vi "POM_PROM_ТЗЧ(3)_host.vi"() -> ()   [LabVIEW 2013]
uses:
  <instrlib>/niDMM/nidmm.llb/niDMM Resolution in Digits.ctl
  <instrlib>/niDMM/nidmm.llb/niDMM Function.ctl
  <vilib>/Analysis/baseanly.llb/Mean (DBL).vi
  <instrlib>/niDMM/nidmm.llb/niDMM Configure Measurement Digits.vi
  <vilib>/Analysis/NI_AALBase.lvlib
  <instrlib>/niDCPower/nidcpower.llb/niDCPower Measurement Type.ctl
panel:
  in  "Нагрев":bool
  in  "В ручную":bool
  in  "Напряжение Пельтье":dbl=0.03
  in  "milliseconds to wait 2":u32=40
  out "Monitor current, uA":dbl(graph)=356.9975233403966
  in  "Порог типатиристора, мА":dbl=55.0
  out "Счетчик сбоев":dbl=6.0
  out "Температура":i32=25
  out "Образец":i32=180201
  out "Сеанс":i32=5
  out "Ион":string="Проверка"
  in  "SEL simulation":bool
  out "refnum out":refnum<file>
  in  "Облучение!":bool
  out "Стабилизировано":bool=TRUE
  in  "+ V TEC для новой точки":dbl=0.11 format="%#_13g"
  in  "Вычет для \"антиразгона\"":dbl format="%#_13g"
  in  "Оставить в раб.\nрежиме":bool
  out "Boolean":bool
  in  "Num_hits_req":u64
  out "Num_hits":u64=15
  in  "Count_hits?":bool
  in  "tstab между точками, мс":u32=1
  in  "Предел тока PDext, мА":dbl=20.0
  in  "Отладка(F)/\n/Рабочий(T)":bool=TRUE
  out "TEC_current, mA":dbl=84.01255498914388
  in  "Param_Log":path=path "D:/#rkm/Фонон-4/ТермоЛазер/Фонон-4_ПОМ_ПрОМ/Прога/Updated/ThermoLaser/Logs/Проверка"
  in  "trelax":u32=35000
  out "Volt_onRes":dbl=2.4602762193630356
  out "NoStab":bool
  out "Operating Current, mA":dbl=48.79715117716259
  in  "Desirable Operating current, mA":dbl=50.0 format="%#_6f"
  in  "Up_Volt_limit":dbl=5.0
  in  "Low_Volt_limit":dbl=1.0
  out "ThRes_stabil":bool=TRUE
  out "Подстроенное напряжение\nстабилизации":dbl=0.22536355468750027
  out "ThRes value":dbl=18041.63984375
  in  "Optimum ThRes":dbl=18000.0 format="%#_6f"
  in  "Предел тока LD, мА":dbl=100.0
  in  "Предел тока ТЕС, мА":dbl=300.0
  in  "Tab Control":enum32{"Page 1", "Page 2", "Page 3", "Page 4"}(tab)=enum."Page 4"
  out "RES(U_TEC) Graph":cluster{dbl[], dbl[]}(graph)={[-0.0, 0.025, 0.05, 0.07500000000000001, 0.1, 0.125, 0.15, 0.175, 0.19999999999999998, 0.22499999999999998, 0.24999999999999997, 0.27499999999999997, 0.3, 0.325, 0.35000000000000003, 0.37500000000000006, 0.4000000000000001, 0.4250000000000001, 0.4500000000000001, 0.47500000000000014, 0.5000000000000001, 0.5250000000000001, 0.5500000000000002, 0.5750000000000002, 0.6000000000000002, 0.6250000000000002, 0.6500000000000002, 0.6750000000000003, 0.7000000000000003, 0.7250000000000003, 0.7500000000000003, 0.7750000000000004], [15319.04365234375, 15328.19267578125, 15358.49169921875, 15409.562109375, 15479.3826171875, 15563.1861328125, 15668.50888671875, 15780.12734375, 15906.40224609375, 16043.244921875, 16186.97255859375, 16341.84609375, 16507.0697265625, 16676.522265625, 16856.963671875, 17044.884375, 17239.0294921875, 17436.3736328125, 17641.744140625, 17850.8728515625, 18071.7896484375, 18291.20625, 18518.965625, 18750.4271484375, 18987.4517578125, 19230.0744140625, 19480.026171875, 19731.8517578125, 19984.940234375, 20249.54140625, 20514.206640625, 20780.055078125]}
  out "RES(I_TEC) Graph":cluster{dbl[], dbl[]}(graph)={[0.03457500435386299, 4.049114950716204, 7.9212407853678135, 11.611043015146826, 15.078954849250364, 18.53827902856892, 21.88408259580828, 25.295266856430793, 28.546483256934756, 31.60504570629327, 34.77027313644012, 37.80993408960394, 40.856486299311584, 43.94949565069024, 47.03219408159836, 50.06845592920464, 52.92926046093485, 55.95350027659507, 58.865931959242474, 61.84202368829837, 64.7802788203752, 67.60156326899994, 70.44177990185035, 73.41963022613506, 76.46974363403558, 79.22741287887104, 82.2001312992484, 85.07135997639818, 88.0785044464861, 90.98931976346292, 93.95691599392462, 96.75420696595256], [15319.04365234375, 15328.19267578125, 15358.49169921875, 15409.562109375, 15479.3826171875, 15563.1861328125, 15668.50888671875, 15780.12734375, 15906.40224609375, 16043.244921875, 16186.97255859375, 16341.84609375, 16507.0697265625, 16676.522265625, 16856.963671875, 17044.884375, 17239.0294921875, 17436.3736328125, 17641.744140625, 17850.8728515625, 18071.7896484375, 18291.20625, 18518.965625, 18750.4271484375, 18987.4517578125, 19230.0744140625, 19480.026171875, 19731.8517578125, 19984.940234375, 20249.54140625, 20514.206640625, 20780.055078125]}
  out "I_PD_Ext(I_LD) Graph":cluster{dbl[], dbl[]}(graph)={[0.0, 5.125820672560687, 10.202363077068034, 15.09070291650038, 20.026524721844005, 24.848748653112324, 29.706585438813228, 34.55255888002156, 39.41379829521783, 44.31743313126964, 49.35841653002704], [0.6213749657825949, 0.6126206411732633, 0.5986137214569519, 0.5846068013204628, 0.5933611264550083, 0.5670981505590477, 0.5355825775341941, 0.586357666360488, 0.5355825775341941, 0.5478386339632713, 0.5390843079753067]}
  out "I_PD(I_LD) Graph":cluster{dbl[], dbl[]}(graph)={[0.0, 5.125820672560687, 10.202363077068034, 15.09070291650038, 20.026524721844005, 24.848748653112324, 29.706585438813228, 34.55255888002156, 39.41379829521783, 44.31743313126964, 49.35841653002704], [0.00446055423708458, 0.1890051237296575, 1.3185992656872259, 47.69851657329127, 96.3842059718445, 145.3466946259141, 195.95923949964345, 243.1108383461833, 288.08951028622687, 334.6654470078647, 377.8655605856329]}
  out "I_pd, uA":dbl
  out "IPD(ext), mA":dbl
  out "V2(I_LD) Graph":cluster{dbl[], dbl[]}(graph)={[0.0, 5.125820672560687, 10.202363077068034, 15.09070291650038, 20.026524721844005, 24.848748653112324, 29.706585438813228, 34.55255888002156, 39.41379829521783, 44.31743313126964, 49.35841653002704], [0.0006418486043783589, 1.1699665507043246, 1.452329111789965, 1.6798119558569469, 1.9201177244634586, 2.150803801269446, 2.3862573437846697, 2.612869753183121, 2.8439823589319366, 3.0683008415602466, 3.3013683877429134]}
  out "Forward Voltage, V":dbl
  out "OP(I_LD) Graph":cluster{dbl[], dbl[]}(graph)={[0.0, 5.125820672560687, 10.202363077068034, 15.09070291650038, 20.026524721844005, 24.848748653112324, 29.706585438813228, 34.55255888002156, 39.41379829521783, 44.31743313126964, 49.35841653002704], [0.0, 0.0, 0.02, 0.74, 1.5, 2.27, 3.0300000000000002, 3.8, 4.58, 5.33, 6.119999999999999]}
  out "Ophir, mW":dbl
  out "Пороговый ток":dbl
  out "ExtPhotodiode Current":dbl(graph)
  out "Boolean 2":bool
  out "Сопротивление терморез-ра":dbl(graph)=16035.80078125
  out "thRes_adj":dbl=16035.80078125 format="%0.2f"
  in  "Source-Ohm w8":u32=1000
  in  "Coeff_High":dbl=90000.0 format="%#_13g"
  in  "Coeff_low":dbl=20000.0 format="%#_13g"
  in  "Coeff_thr":dbl=1500.0
  out "+Voltage\nrequired":dbl=0.0008410915798611111
  out "Разница ThRes":dbl=75.6982421875
  out "Operating Current":dbl(graph)
  out "Готовы облучать":bool
  out "accommodated voltage (out)":dbl=5.873393180232852
  in  "4070_Rele_source":enum16{"S2_Ch0", "S1_Ch2"}(ring)
  in  "the upper limit for the voltage_LD":dbl=6.0
  in  "the lower limit for the voltage_LD":dbl=1.0
  in  "Start voltage_LD":dbl=2.0 format="%#.7f"
  in  "accuracy_LD":dbl=0.09999999999999999 step=0.01
  in  "Res_LD":dbl=50.0
  in  "TEC_Source":enum16{"S1_Ch2", "S2_Ch0", "S3_Ch1"}(ring)
  in  "Start voltage":dbl=0.1 format="%#.7f"
  in  "the upper limit for the voltage":dbl=0.9
  in  "the lower limit for the voltage":dbl
  in  "Точность ThRes":dbl=75.0 step=0.01
  out "Ro, Ом":dbl=15321.56484375
  in  "OphirLMMeasurementLib.ICoLMMeasurement":refnum<k7>
  out "hDevice":i32=1004
  out "Ophir_address":refnum<k7>
  in  "Power Enable":bool
  in  "4071(2)":refnum<k15>
  out "4071(2)_adress":refnum<k15>="PXI1Slot4_2 (12)" caption="4071(1)_out"
  in  "4071(1)":refnum<k15>="PXI1Slot5_2"
  out "4071(1)_adress":refnum<k15>="PXI1Slot5_2 (8)" caption="4071(1)_out"
  out "4070_address":refnum<k15>="PXI1Slot4_2 (8)" caption="4070_out"
  in  "4070":refnum<k15>="PXI1Slot6_3"
  in  "Source_3":refnum<k15>
  out "Source_3_Vcc_out":refnum<k15> caption="S_3_out"
  out "Source_2_Vcc_out":refnum<k15>="PXI1Slot6" caption="S_2_out"
  in  "Source_2":refnum<k15>="PXI1Slot3"
  out "Source_1_Vcc_out":refnum<k15>="PXI1Slot2_2" caption="S_1_out"
  in  "Source_1":refnum<k15>="PXI1Slot2_2"
  out "Прервать":bool=TRUE
  in  "milliseconds to wait":u32=2000
  in  "Шаг напр\nдля TEC, В":dbl=0.025
  in  "Начальное\nнапряжение TEC, В":dbl
  in  "кол-во точек для TEC":i32=32
  in  "stop":bool
  in  "Case":T1(ring)=enum."Quit"
  out "Выполняется":bool
  in  "Раб. режим LD":bool
  in  "Хар-ка TEC":bool
  in  "Хар-ки от I_LD":bool
  out "Status:":string="IDLE"
  out "Подстроенный ток, mA":dbl=48.878464927379845
  in  "Шаг, мА":dbl=5.0
  in  "Начальный ток, мА":dbl
  in  "Кол-во точек":i32=11
  # "20"
  # "7"
  # "5"
  # "ток Пельтье во время стабилизации"
  # "0,15"
  # "Охлаждение"
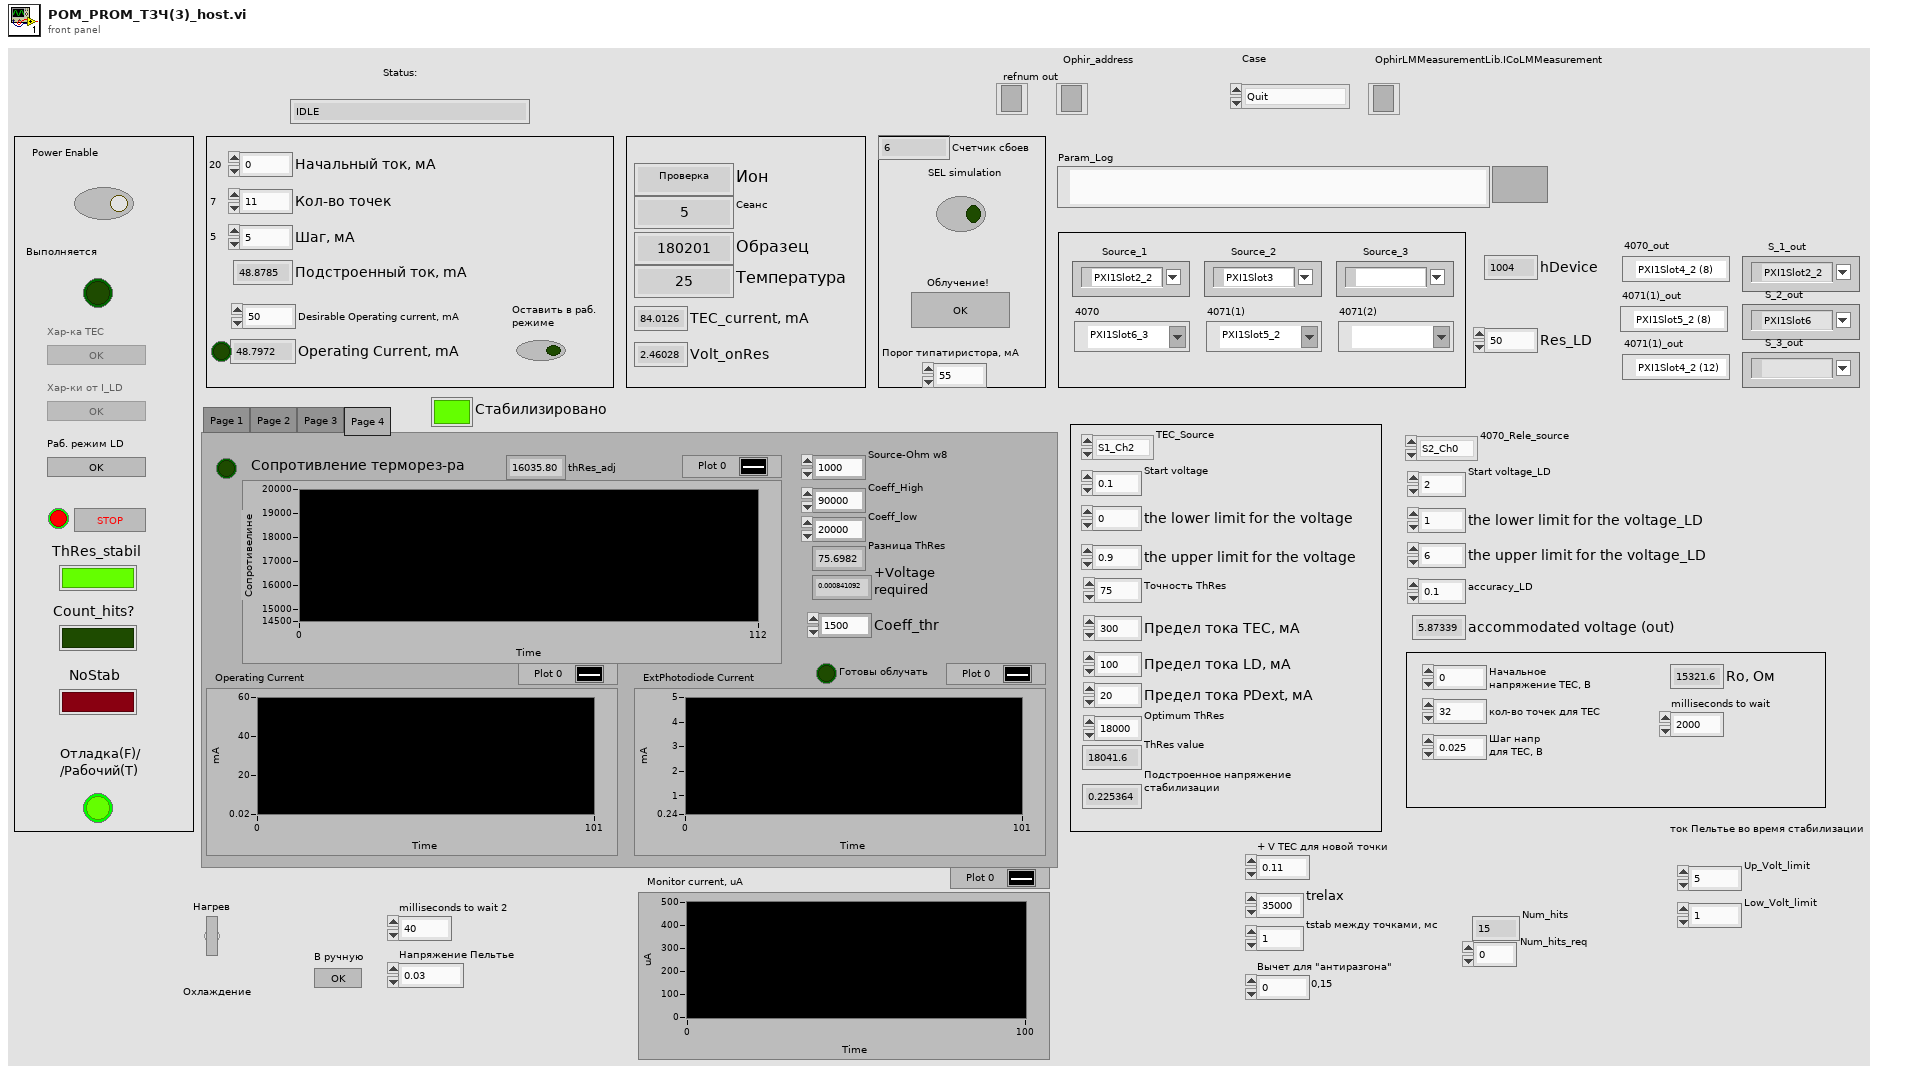
[diagram p1: front panel]
types:
  T1 = enum16{"Initialization", "TEC_Chars", "TRes_Check(Idle)", "Characteristics", "Bias", "Quit"}
  T2 = typedef "niDMM Function.ctl" = enum16{"DC Volts", "AC Volts", "DC Current", "AC Current", "2-wire Resistance", "4-wire Resistance", "Diode", "Frequency", "Period", "AC Volts DC Coupled", "Capacitance", "Inductance", "Temperature"}
  T3 = enum8{"Enabled", "Disabled", "Disabled and Grayed Out"}
  T4 = typedef "niDMM Resolution in Digits.ctl" = dbl
  T5 = enum16{"open", "replace", "create", "open or create", "replace or create", "replace or create with confirmation"}
  T6 = typedef "niDCPower Measurement Type.ctl" = i32
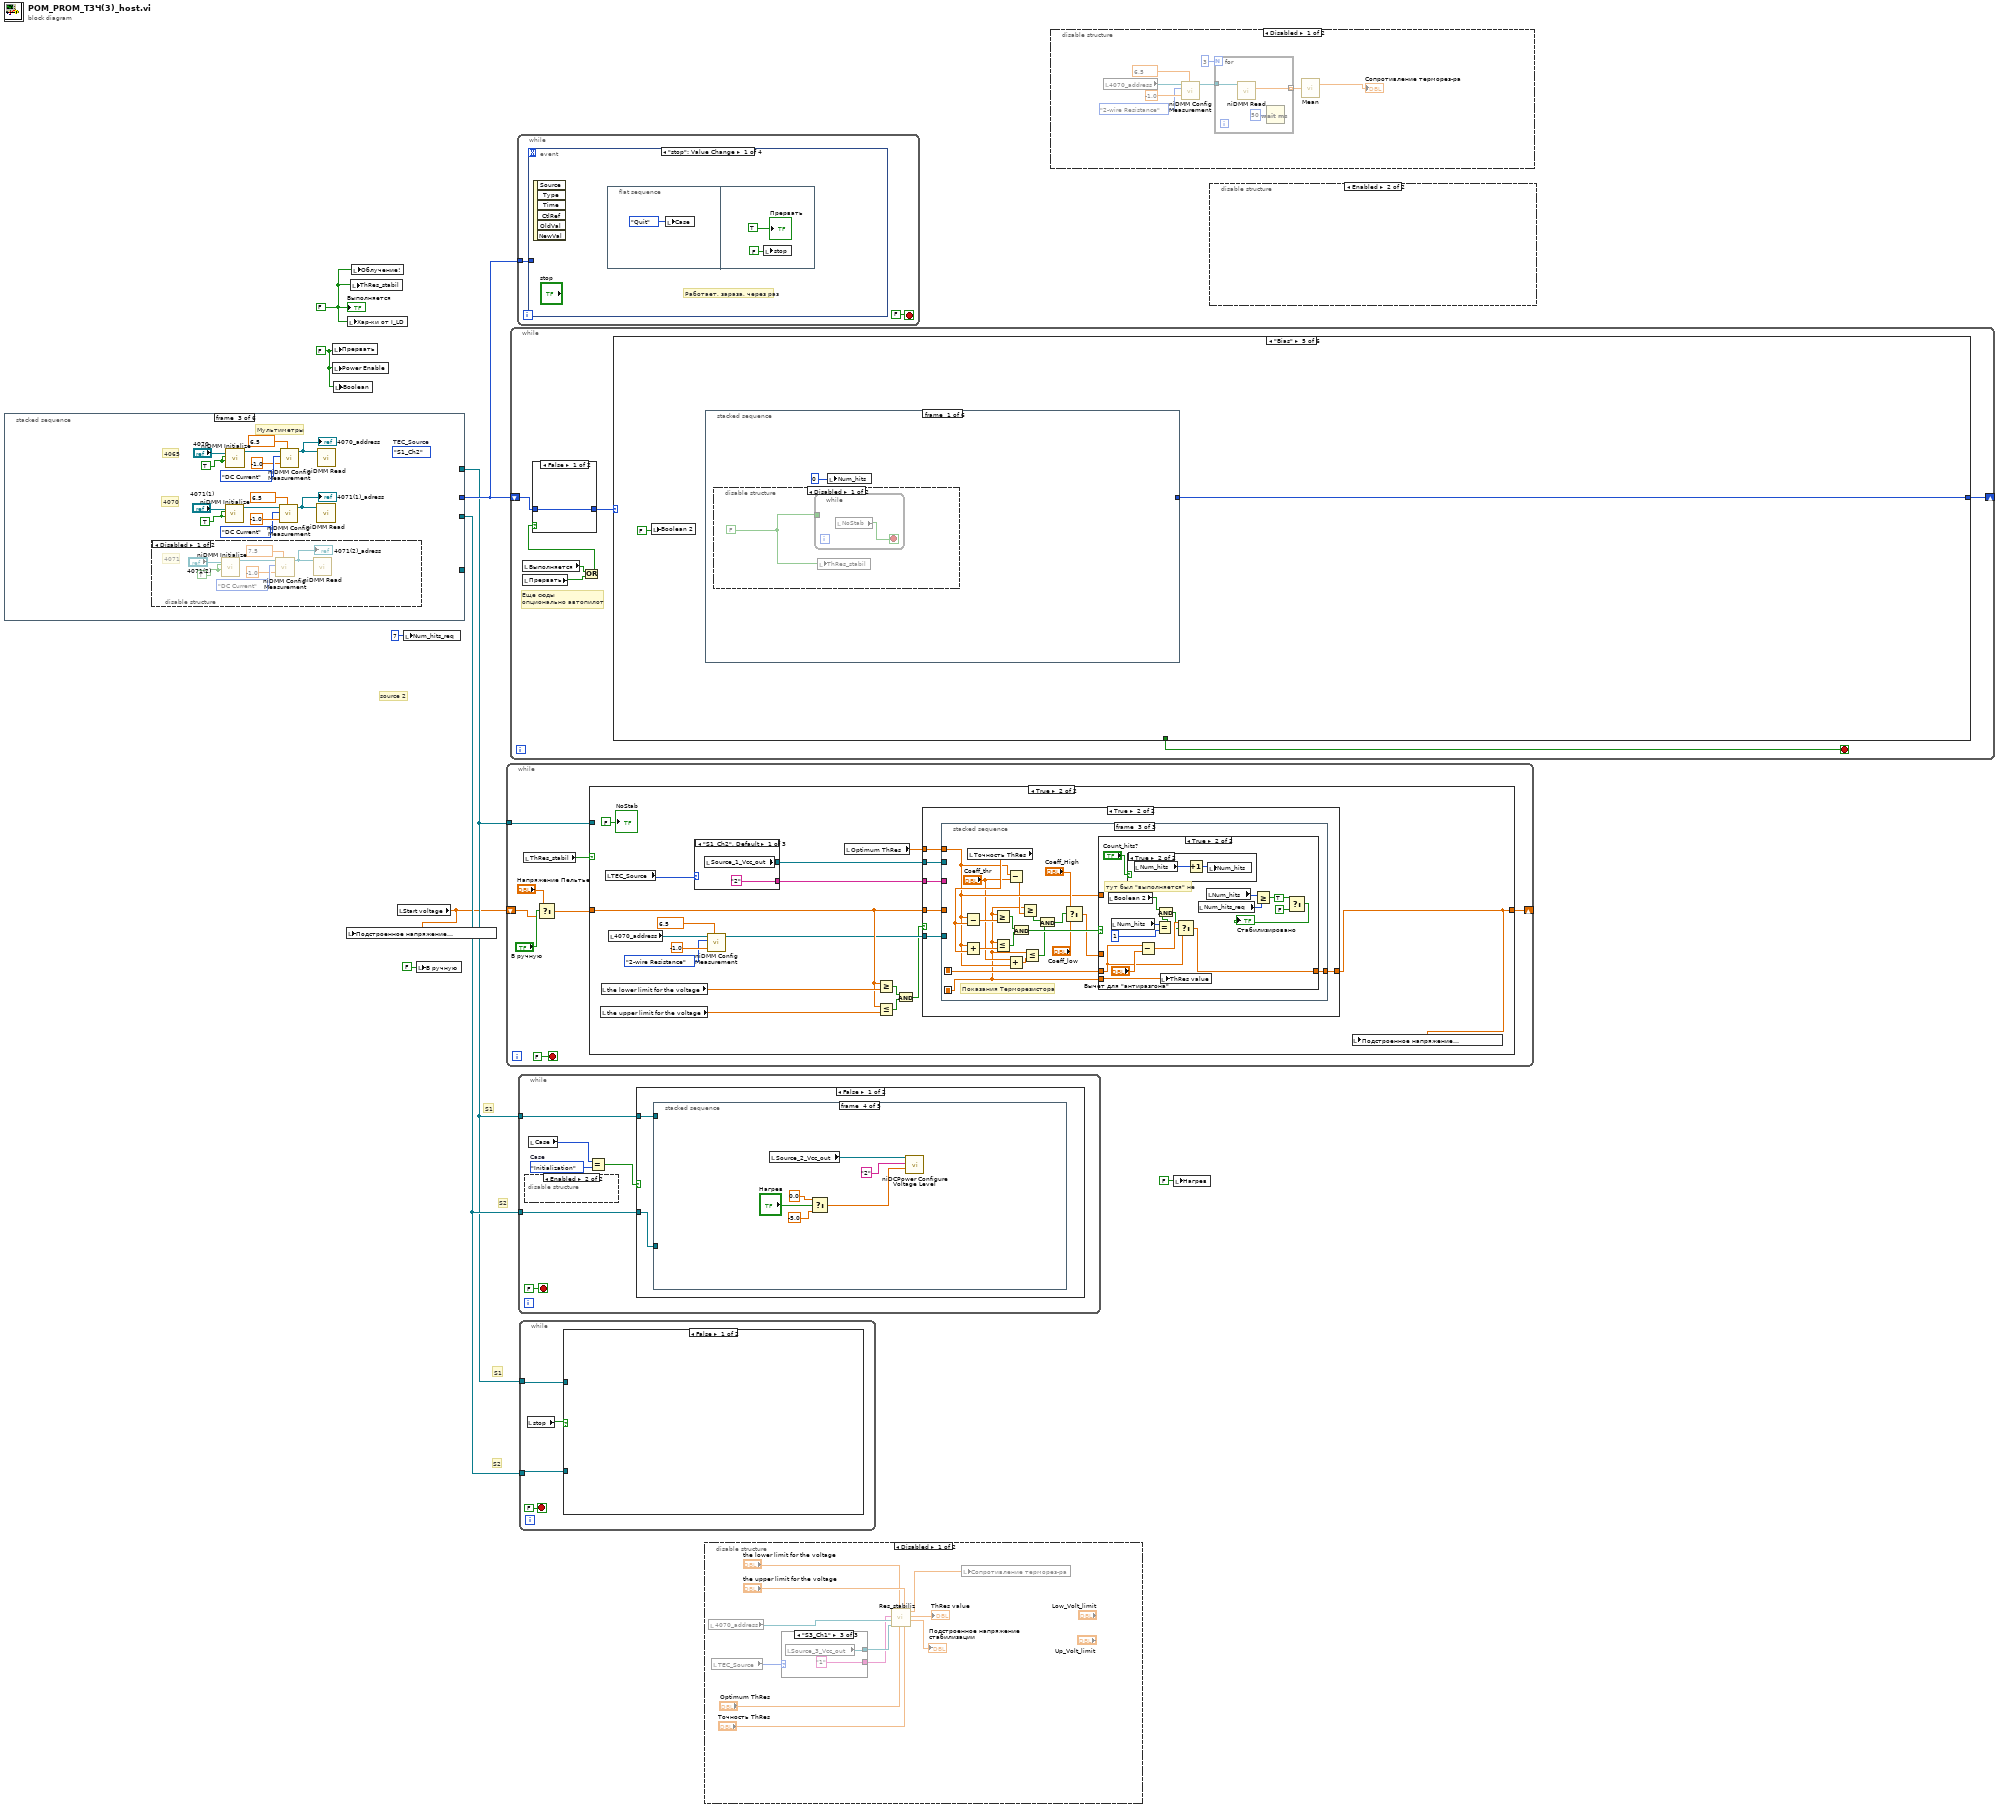
[diagram p0: block diagram]
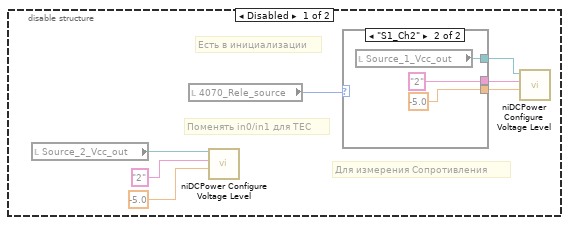
[diagram p3: hidden frame]
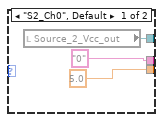
[diagram p4: hidden frame]
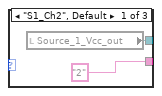
[diagram p5: hidden frame]
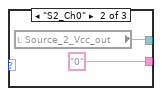
[diagram p6: hidden frame]
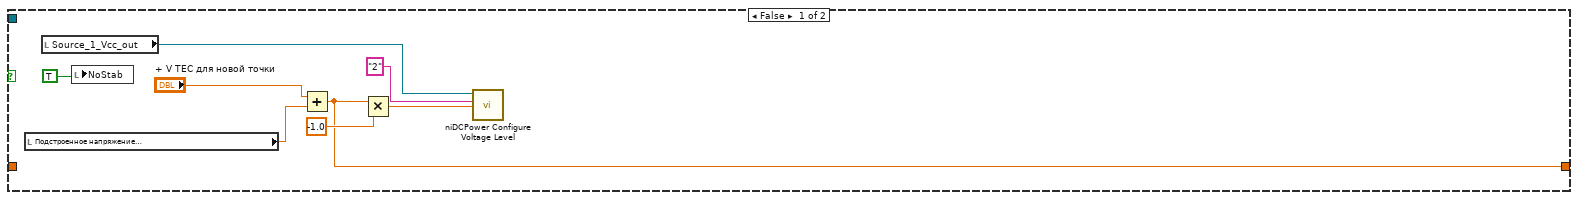
[diagram p8: hidden frame]
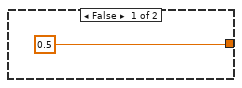
[diagram p9: hidden frame]
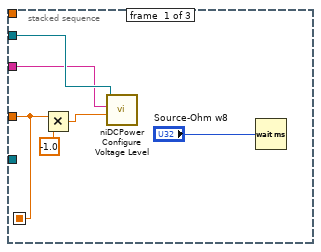
[diagram p10: hidden frame]
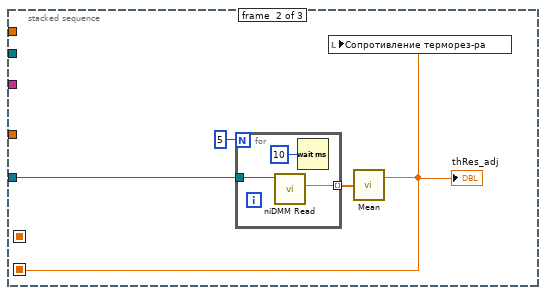
[diagram p11: hidden frame]
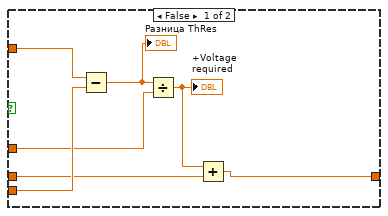
[diagram p12: hidden frame]
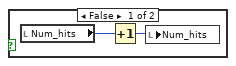
[diagram p13: hidden frame]
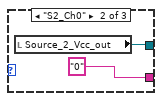
[diagram p14: hidden frame]
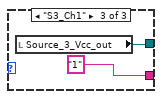
[diagram p15: hidden frame]
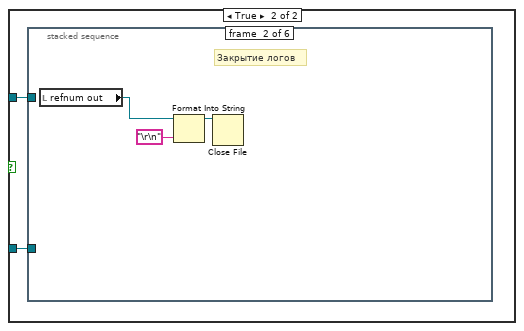
[diagram p16: hidden frame]
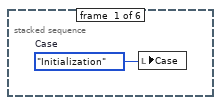
[diagram p17: hidden frame]
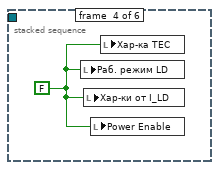
[diagram p19: hidden frame]
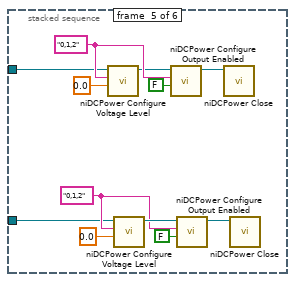
[diagram p20: hidden frame]
diagram:
  w4 = FALSE
  w6 = FALSE
  # "source 2"
  # "S1"
  # "S2"
  # "S2"
  # "S1"
  n1 = stacked-sequence {
    tunnel: [_ _ _ _ _ w93] -> w9
    tunnel: [_ w20 _ _ _ _] -> w8
    tunnel: [_ w19 _ _ _ _] -> w7
    tunnel: [_ w18 _ _ _ _] -> _
    frame #0 {
      n2 = while {
        stop <- w16 stop-if-true
        w11 = T3."Disabled and Grayed Out" ("Disabled")
        n3 = local write "Стабилизировано"(FALSE) -> ()
        n4 = property on="Хар-ка TEC" class="Bool (strict)"("DisabledEnum"=w11) -> ()  [unwired: 2 in, 2 out]
        n5 = property on="Раб. режим LD" class="Bool (strict)"("DisabledEnum"=w11) -> ()  [unwired: 2 in, 2 out]
        n6 = property on="Хар-ки от I_LD" class="Bool (strict)"("DisabledEnum"=w11) -> ()  [unwired: 2 in, 2 out]
        n7 = local write "Status:"("Ожидание Power Enable" ("Status:")) -> ()
        n8 = local read "stop"() -> (w14:bool)
        n9 = case shown="True" w14 {
          frame False {
          }
          frame True {
            n10 = local write "Прервать"(TRUE) -> ()
          }
        }
        n11 = Or(x=w14, y="Power Enable") -> (x .or. y?=w16:bool)
        n12 = Wait (ms)(milliseconds to wait=u32 100) -> ()  [unwired: 1 out]
      }
    }
    frame #1 {
      # "Источники"
      n13 = disable-structure shown="Disabled" {
        disable-tunnel: [w41 _] -> w18
        frame Disabled {
          n14 = call <instrlib>:"niDCPower Initialize.vi"("resource name"="Source_3") -> ("instrument handle out"=w45:refnum<k15>)  [unwired: 3 in, 7 out]
          n15 = call <instrlib>:"niDCPower Configure Voltage Level.vi"("voltage level"=0.0, "channel name"="0", "instrument handle"=w45) -> ("instrument handle out"=w44:refnum<k15>)  [unwired: 7 in, 1 out]
          n16 = call <instrlib>:"niDCPower Configure Voltage Level.vi"("voltage level"=0.0, "channel name"="1", "instrument handle"=w44) -> ("instrument handle out"=w50:refnum<k15>)  [unwired: 7 in, 1 out]
          n17 = call <instrlib>:"niDCPower Configure Voltage Level.vi"("voltage level"=0.0, "channel name"="2", "instrument handle"=w50) -> ("instrument handle out"=w41:refnum<k15>)  [unwired: 7 in, 1 out]
          "Source_3_Vcc_out" <- w41
        }
        frame Enabled {
        }
      }
      n18 = call <instrlib>:"niDCPower Initialize.vi"("resource name"="Source_1") -> ("instrument handle out"=w34:refnum<k15>)  [unwired: 3 in, 7 out]
      n19 = call <instrlib>:"niDCPower Initialize.vi"("resource name"="Source_2") -> ("instrument handle out"=w27:refnum<k15>)  [unwired: 3 in, 7 out]
      n20 = call <instrlib>:"niDCPower Configure Voltage Level.vi"("voltage level"=0.0, "channel name"="0", "instrument handle"=w34) -> ("instrument handle out"=w33:refnum<k15>)  [unwired: 7 in, 1 out]
      n21 = call <instrlib>:"niDCPower Configure Voltage Level.vi"("voltage level"=0.0, "channel name"="0", "instrument handle"=w27) -> ("instrument handle out"=w28:refnum<k15>)  [unwired: 7 in, 1 out]
      n22 = call <instrlib>:"niDCPower Configure Voltage Level.vi"("voltage level"=0.0, "channel name"="1", "instrument handle"=w33) -> ("instrument handle out"=w40:refnum<k15>)  [unwired: 7 in, 1 out]
      n23 = call <instrlib>:"niDCPower Configure Voltage Level.vi"("voltage level"=0.0, "channel name"="1", "instrument handle"=w28) -> ("instrument handle out"=w22:refnum<k15>)  [unwired: 7 in, 1 out]
      n24 = call <instrlib>:"niDCPower Configure Voltage Level.vi"("voltage level"=0.0, "channel name"="2", "instrument handle"=w40) -> ("instrument handle out"=w19:refnum<k15>)  [unwired: 7 in, 1 out]
      "Source_1_Vcc_out" <- w19
      n25 = call <instrlib>:"niDCPower Configure Voltage Level.vi"("voltage level"=0.0, "channel name"="2", "instrument handle"=w22) -> ("instrument handle out"=w20:refnum<k15>)  [unwired: 7 in, 1 out]
      "Source_2_Vcc_out" <- w20
    }
    frame #2 {
      w52 = T4 6.5 items=["3 1/2"=3.5, "4 1/2"=4.5, "5 1/2"=5.5, "6 1/2"=6.5, "7 1/2"=7.5] ("Resolution in Digits")
      w54 = TRUE ("Reset")
      (unwired) enum16{"S1_Ch2", "S2_Ch0", "S3_Ch1"}."S1_Ch2"  # TEC_Source
      w65 = T4 6.5 items=["3 1/2"=3.5, "4 1/2"=4.5, "5 1/2"=5.5, "6 1/2"=6.5, "7 1/2"=7.5] ("Resolution in Digits")
      w63 = TRUE ("Reset")
      # "4065"
      # "4070"
      # "Мультиметры"
      n26 = disable-structure shown="Disabled" {
        frame Disabled {
          w72 = T4 7.5 items=["3 1/2"=3.5, "4 1/2"=4.5, "5 1/2"=5.5, "6 1/2"=6.5, "7 1/2"=7.5] ("Resolution in Digits")
          w70 = TRUE ("Reset")
          # "4071"
          n27 = call <instrlib>:"niDMM Initialize.vi"("Reset"=w70, "ID Query"=w70, "Instrument Descriptor"="4071(2)") -> ("instrument handle out"=w68:refnum<k15>)  [unwired: 7 in, 1 out]
          n28 = call-poly <instrlib>:"niDMM Config Measurement.vi"("Range"=-1.0 ("Configuration:Measurement Options:Max Frequency"), "Resolution in Digits"=w72, "Function"=niDMM_Function."DC Current" ("multimeter mode"), "instrument handle"=w68) -> ("instrument handle out"=w66:refnum<k15>)  [unwired: 6 in, 1 out]
          "4071(2)_adress" <- w66
          n29 = call <instrlib>:"niDMM Read.vi"("instrument handle"=w66) -> ()  [unwired: 8 in, 3 out]
        }
        frame Enabled {
        }
      }
      n30 = call <instrlib>:"niDMM Initialize.vi"("Reset"=w54, "ID Query"=w54, "Instrument Descriptor"="4071(1)") -> ("instrument handle out"=w56:refnum<k15>)  [unwired: 7 in, 1 out]
      n31 = call <instrlib>:"niDMM Initialize.vi"("Reset"=w63, "ID Query"=w63, "Instrument Descriptor"="4070") -> ("instrument handle out"=w61:refnum<k15>)  [unwired: 7 in, 1 out]
      n32 = call-poly <instrlib>:"niDMM Config Measurement.vi"("Range"=-1.0 ("Configuration:Measurement Options:Max Frequency"), "Resolution in Digits"=w52, "Function"=niDMM_Function."DC Current" ("multimeter mode"), "instrument handle"=w56) -> ("instrument handle out"=w58:refnum<k15>)  [unwired: 6 in, 1 out]
      "4071(1)_adress" <- w58
      n33 = call-poly <instrlib>:"niDMM Config Measurement.vi"("Range"=-1.0 ("Configuration:Measurement Options:Max Frequency"), "Resolution in Digits"=w65, "Function"=niDMM_Function."DC Current" ("multimeter mode"), "instrument handle"=w61) -> ("instrument handle out"=w59:refnum<k15>)  [unwired: 6 in, 1 out]
      "4070_address" <- w59
      n34 = call <instrlib>:"niDMM Read.vi"("instrument handle"=w58) -> ()  [unwired: 8 in, 3 out]
      n35 = call <instrlib>:"niDMM Read.vi"("instrument handle"=w59) -> ()  [unwired: 8 in, 3 out]
    }
    frame #3 {
      n36 = disable-structure shown="Disabled" {
        frame Disabled {
          n37 = Automation Open(Automation Refnum="OphirLMMeasurementLib.ICoLMMeasurement") -> (Automation Refnum=w81:refnum<k7>)  [unwired: 3 in, 1 out]
          n38 = invoke class="ICoLMMeasurement" method="ScanUSB"(reference=w81) -> (reference out=w83:refnum<k7>, "serialNumbers"=w80:variant)  [unwired: 3 in, 2 out]
          "Ophir_address" <- w83
          n39 = Variant To Data(type=string[] [], Variant=w80) -> (data=w79:string[])  [unwired: 1 in, 1 out]
          n40 = Index Array(array=w79, index=0) -> (element=w76:string)
          n41 = invoke class="ICoLMMeasurement" method="OpenUSBDevice"(reference=w83, "serialNumber"=w76) -> (reference out=w75:refnum<k7>, "hDevice"=w74:i32)  [unwired: 3 in, 3 out]
          "hDevice" <- w74
          n42 = invoke class="ICoLMMeasurement" method="StartStream"(reference=w75, "hDevice"=w74, "channel"=0) -> ()  [unwired: 2 in, 5 out]
        }
        frame Enabled {
        }
      }
    }
    frame #4 {
      n43 = while {
        stop <- w85 stop-if-true
        n44 = call "Save_dialogue_number_ION.vi"() -> ("Температура 2"=→"Температура":i32, "Номер образца 2"=→"Образец":i32, "Номер сеанса 2"=→"Сеанс":i32, "Ион 2"=→"Ион":string, "OK Button 2"=w85:bool)  [unwired: 5 in]
        n45 = Wait (ms)(milliseconds to wait=u32 250) -> ()  [unwired: 1 out]
      }
      "Счетчик сбоев" <- 0.0
    }
    frame #5 {
      (unwired) enum16{"S2_Ch0", "S1_Ch2"}."S2_Ch0"  # 4070_Rele_source
      w93 = T1."Initialization"  # Case
      n46 = property on="Сопротивление терморез-ра" class="WFChart (strict)"("History Data"=dbl[] []) -> ()  [unwired: 2 in, 2 out]
      n47 = local write "Start voltage"("Start voltage") -> ()
    }
  }
  n48 = local write "Прервать"(w6) -> ()
  n49 = local write "Power Enable"(w6) -> ()
  n50 = local write "Boolean"(w6) -> ()
  n51 = local write "Хар-ки от I_LD"(w4) -> ()
  n52 = local write "ThRes_stabil"(w4) -> ()
  n53 = local write "Облучение!"(w4) -> ()
  n54 = local read "Start voltage"() -> (w5:dbl)
  n55 = local write "Подстроенное напряжение\nстабилизации"(w5) -> ()
  n56 = local write "Num_hits_req"(u64 7 ("Num_hits_req")) -> ()
  n57 = local write "В ручную"(FALSE ("В ручную")) -> ()
  n58 = while {
    shift-right: [w99] -> _
    shift-left: w5 -> [w95]
    tunnel: w7 -> [w98]
    stop <- FALSE stop-if-true
    n59 = local read "ThRes_stabil"() -> (w100:bool)
    n60 = Select(t="Напряжение Пельтье", s="В ручную", f=w95) -> (s? t:f=w94:dbl)
    n61 = case shown="True" w100 {
      tunnel: [w103 w115] -> w99
      tunnel: w94 -> [_ w121]
      tunnel: w98 -> [_ _]
      frame False {
        n62 = local read "Подстроенное напряжение\nстабилизации"() -> (w102:dbl)
        n63 = local read "Source_1_Vcc_out"() -> (w107:refnum<k15>)
        n64 = local write "NoStab"(TRUE) -> ()
        n65 = Add(x="+ V TEC для новой точки", y=w102) -> (x+y=w103:dbl)
        n66 = Multiply(x=w103, y=-1.0) -> (x*y=w104:dbl)
        n67 = call <instrlib>:"niDCPower Configure Voltage Level.vi"("voltage level"=w104, "channel name"="2", "instrument handle"=w107) -> ()  [unwired: 7 in, 2 out]
      }
      frame True {
        w117 = T4 6.5 items=["3 1/2"=3.5, "4 1/2"=4.5, "5 1/2"=5.5, "6 1/2"=6.5, "7 1/2"=7.5] ("Resolution in Digits")
        n68 = local read "the upper limit for the voltage"() -> (w122:dbl)
        n69 = local read "the lower limit for the voltage"() -> (w123:dbl)
        n70 = local read "TEC_Source"() -> (w124:enum16{"S1_Ch2", "S2_Ch0", "S3_Ch1"})
        n71 = local read "4070_address"() -> (w116:refnum<k15>)
        n72 = case shown="\"S1_Ch2\", Default" w124 {
          tunnel: [w195 w197 w199] -> w126
          tunnel: ["2" "0" "1"] -> w125
          frame "S1_Ch2", Default {
            n73 = local read "Source_1_Vcc_out"() -> (w195:refnum<k15>)
          }
          frame "S2_Ch0" {
            n74 = local read "Source_2_Vcc_out"() -> (w197:refnum<k15>)
          }
          frame "S3_Ch1" {
            n75 = local read "Source_3_Vcc_out"() -> (w199:refnum<k15>)
          }
        }
        n76 = call-poly <instrlib>:"niDMM Config Measurement.vi"("Range"=-1.0 ("Configuration:Measurement Options:Max Frequency"), "Resolution in Digits"=w117, "Function"=niDMM_Function."2-wire Resistance" ("multimeter mode"), "instrument handle"=w116) -> ("instrument handle out"=w114:refnum<k15>)  [unwired: 6 in, 1 out]
        n77 = local read "Optimum ThRes"() -> (w110:dbl)
        n78 = Greater Or Equal?(x=w121, y=w123) -> (x >= y?=w113:bool)
        n79 = Less Or Equal?(x=w121, y=w122) -> (x <= y?=w112:bool)
        n80 = And(x=w113, y=w112) -> (x .and. y?=w111:bool)
        n81 = case shown="True" w111 {
          tunnel: w121 -> [_ w131]
          tunnel: w126 -> [_ w133]
          tunnel: w125 -> [_ w132]
          tunnel: w110 -> [_ w129]
          tunnel: w114 -> [_ w130]
          tunnel: [0.5 w128] -> w115
          frame False {
          }
          frame True {
            n82 = stacked-sequence {
              seq-local: [w134 _ _] -> [_ _ w160]
              seq-local: [_ w141 _] -> [_ _ w151]
              tunnel: w133 -> [w139 _ _]
              tunnel: w132 -> [w138 _ _]
              tunnel: w131 -> [w134 _ _]
              tunnel: w130 -> [_ w140 _]
              tunnel: w129 -> [_ _ w154]
              tunnel: [_ _ w159] -> w128
              frame #0 {
                n83 = Multiply(x=w134, y=-1.0) -> (x*y=w135:dbl)
                n84 = call <instrlib>:"niDCPower Configure Voltage Level.vi"("voltage level"=w135, "channel name"=w138, "instrument handle"=w139) -> ()  [unwired: 7 in, 2 out]
                n85 = Wait (ms)(milliseconds to wait="Source-Ohm w8") -> ()  [unwired: 1 out]
              }
              frame #1 {
                n86 = for {
                  N: 5 -> [_]
                  tunnel: w140 -> [w146]
                  tunnel: [w145] -> w142 mode=indexing
                  n87 = call <instrlib>:"niDMM Read.vi"("instrument handle"=w146) -> ("Measurement"=w145:dbl)  [unwired: 8 in, 2 out]
                  n88 = Wait (ms)(milliseconds to wait=u32 10) -> ()  [unwired: 1 out]
                }
                n89 = call-poly <vilib>:"Mean.vi"("X"=w142) -> ("mean"=w141:dbl)  [unwired: 1 out]
                "thRes_adj" <- w141
                n90 = local write "Сопротивление терморез-ра"(w141) -> ()
              }
              frame #2 {
                # "Показания Терморезистора"
                n91 = local read "Точность ThRes"() -> (w158:dbl)
                n92 = Subtract(x=w154, y=w158) -> (x-y=w163:dbl)
                n93 = Add(x=w154, y=w158) -> (x+y=w164:dbl)
                n94 = Greater Or Equal?(x=w151, y=w163) -> (x >= y?=w165:bool)
                n95 = Less Or Equal?(x=w151, y=w164) -> (x <= y?=w162:bool)
                n96 = Subtract(x=w154, y="Coeff_thr") -> (x-y=w152:dbl)
                n97 = Add(x="Coeff_thr", y=w154) -> (x+y=w150:dbl)
                n98 = And(x=w165, y=w162) -> (x .and. y?=w161:bool)
                n99 = Greater Or Equal?(x=w151, y=w152) -> (x >= y?=w149:bool)
                n100 = Less Or Equal?(x=w151, y=w150) -> (x <= y?=w148:bool)
                n101 = And(x=w149, y=w148) -> (x .and. y?=w147:bool)
                n102 = Select(t="Coeff_High", s=w147, f="Coeff_low") -> (s? t:f=w155:dbl)
                n103 = case shown="True" w161 {
                  tunnel: [w167 w182] -> w159
                  tunnel: w160 -> [w169 w183]
                  tunnel: w151 -> [w170 w189]
                  tunnel: w154 -> [w171 _]
                  tunnel: w155 -> [w166 _]
                  frame False {
                    n104 = Subtract(x=w171, y=w170) -> (x-y=w172:dbl)
                    "Разница ThRes" <- w172
                    n105 = Divide(x=w172, y=w166) -> (x/y=w168:dbl)
                    "+Voltage\nrequired" <- w168
                    n106 = Add(x=w168, y=w169) -> (x+y=w167:dbl)
                  }
                  frame True {
                    # "тут был \"выполняется\" не"
                    n107 = local read "Boolean 2"() -> (w173:bool)
                    n108 = local read "Num_hits"() -> (w187:u64)
                    n109 = case shown="True" "Count_hits?" {
                      frame False {
                        n110 = local read "Num_hits"() -> (w190:u64)
                        n111 = Increment(x=w190) -> (x+1=w191:u64)
                        n112 = local write "Num_hits"(w191) -> ()
                      }
                      frame True {
                        n113 = local read "Num_hits"() -> (w193:u64)
                        n114 = Increment(x=w193) -> (x+1=w192:u64)
                        n115 = local write "Num_hits"(w192) -> ()
                      }
                    }
                    n116 = Subtract(x=w183, y="Вычет для \"антиразгона\"") -> (x-y=w184:dbl)
                    n117 = Equal?(x=w187, y=1) -> (x = y?=w181:bool)
                    n118 = And(x=w173, y=w181) -> (x .and. y?=w180:bool)
                    n119 = local write "ThRes value"(w189) -> ()
                    n120 = Select(t=w184, s=w180, f=w183) -> (s? t:f=w182:dbl)
                    n121 = local read "Num_hits_req"() -> (w178:u64)
                    n122 = local read "Num_hits"() -> (w179:u64)
                    n123 = Greater Or Equal?(x=w179, y=w178) -> (x >= y?=w177:bool)
                    n124 = Select(t=TRUE, s=w177, f=FALSE) -> (s? t:f=→"Стабилизировано":bool)
                  }
                }
              }
            }
          }
        }
        n125 = local write "Подстроенное напряжение\nстабилизации"(w115) -> ()
        "NoStab" <- FALSE ("NoStab")
      }
    }
  }
  n126 = while {
    shift-right: [w200] -> _
    shift-left: w9 -> [w206]
    stop <- w204 stop-if-true
    # "Еще сюды\nопционально автопилот"
    n127 = local read "Выполняется"() -> (w203:bool)
    n128 = local read "Прервать"() -> (w202:bool)
    n129 = Or(x=w203, y=w202) -> (x .or. y?=w201:bool)
    n130 = case shown="False" w201 {
      tunnel: w206 -> [w207 _]
      tunnel: [w207 "Case"] -> w205
      frame False {
      }
      frame True {
      }
    }
    n131 = case shown="\"Bias\"" w205 {
      tunnel: [_ _ _ _ _ TRUE] -> w204
      tunnel: [w209 w277 w434 w482 w765 T1."Quit" ("Case")] -> w200
      frame "Initialization", Default {
        n132 = stacked-sequence {
          tunnel: [_ _ _ _ T1."TRes_Check(Idle)" ("Case")] -> w209
          frame #0 {
            n133 = property on="Раб. режим LD" class="Bool (strict)"("DisabledEnum"=T3."Enabled" ("Disabled")) -> ()  [unwired: 2 in, 2 out]
          }
          frame #1 {
            # "Питание внешнего фотодиода"
            # "Поменять in0/in1 для ТЕС"
            # "Режим омметра"
            n134 = local read "4070_Rele_source"() -> (w219:enum16{"S2_Ch0", "S1_Ch2"})
            n135 = local read "Source_2_Vcc_out"() -> (w213:refnum<k15>)
            n136 = case shown="\"S2_Ch0\", Default" w219 {
              tunnel: [5.0 -5.0] -> w220
              tunnel: ["0" "2"] -> w221
              tunnel: [w223 w226] -> w222
              frame "S2_Ch0", Default {
                n137 = local read "Source_2_Vcc_out"() -> (w223:refnum<k15>)
              }
              frame "S1_Ch2" {
                n138 = local read "Source_1_Vcc_out"() -> (w226:refnum<k15>)
              }
            }
            n139 = call <instrlib>:"niDCPower Configure Voltage Level.vi"("voltage level"=-5.0, "channel name"="2", "instrument handle"=w213) -> ()  [unwired: 7 in, 2 out]
            n140 = call <instrlib>:"niDCPower Configure Voltage Level.vi"("voltage level"=5.0, "channel name"="1", "instrument handle"=w213) -> ()  [unwired: 7 in, 2 out]
            n141 = call <instrlib>:"niDCPower Configure Voltage Level.vi"("voltage level"=w220, "channel name"=w221, "instrument handle"=w222) -> ()  [unwired: 7 in, 2 out]
            n142 = Wait (ms)(milliseconds to wait=u32 500) -> ()  [unwired: 1 out]
          }
          frame #2 {
            w231 = FALSE
            n143 = local write "NoStab"(w231) -> ()
            n144 = local write "Count_hits?"(w231) -> ()
            n145 = local write "Num_hits"(u64 0 ("Num_hits")) -> ()
            "ThRes_stabil" <- TRUE
            "Boolean 2" <- TRUE
          }
          frame #3 {
            w269 = "\t"
            n146 = local read "Образец"() -> (w249:i32)
            n147 = local read "Температура"() -> (w245:i32)
            n148 = local read "Сеанс"() -> (w240:i32)
            n149 = local read "Ион"() -> (w255:string)
            n150 = Number To Fractional String(number=w249, width (-)=i16 1, precision (6)=i16 0) -> (F-format string=w248:string)  [unwired: 1 in]
            n151 = Number To Fractional String(number=w240, width (-)=i16 1, precision (6)=i16 0) -> (F-format string=w241:string)  [unwired: 1 in]
            n152 = Number To Fractional String(number=w245, width (-)=i16 1, precision (6)=i16 0) -> (F-format string=w244:string)  [unwired: 1 in]
            n153 = Build Path(base path="Param_Log", name or relative path=w255) -> (appended path=w236:path)
            n154 = Build Path(base path=w236, name or relative path="SEL") -> (appended path=w238:path)
            n155 = Concatenate Strings(w248, "_T=" ("string"), w244, "_сеанс" ("string"), w241, ".log" ("string")) -> (w235:string)
            n156 = call <vilib>:"Check if File or Folder Exists.vi"("path"=w238) -> ("file or folder exists?"=w260:bool, "dup path"=w259:path)  [unwired: 8 in, 1 out]
            n157 = case shown="False" w260 {
              tunnel: w259 -> [w274 w275]
              tunnel: [w273 w275] -> w258
              frame False {
                n158 = Create Folder(path (use dialog)=w274) -> (created path=w273:path)  [unwired: 2 in, 2 out]
              }
              frame True {
              }
            }
            n159 = Build Path(base path=w258, name or relative path=w235) -> (appended path=w257:path)
            n160 = Open/Create/Replace File(file path (use dialog)=w257, operation (0:open)=T5."open or create", access (0:read/write)=enum16{"read/write", "read-only", "write-only"}."read/write") -> (refnum out=w239:refnum<file>)  [unwired: 3 in, 2 out]
            n161 = Set File Position(refnum=w239, from (0:start)=enum16{"start", "end", "current"}."end") -> (refnum out=w233:refnum<file>)  [unwired: 2 in, 1 out]
            "refnum out" <- w233
            n162 = Format Into String(initial string=w233, "Time" ("input 1"), w269, "Op_Cur, mA " ("input 6"), w269, "Ipd(EXT), mA", w269, "Im, uA" ("input 6"), w269, "Облучение?", w269, "Превышение тока?", "\r\n") -> (resulting string=w270:refnum<file>)  [unwired: 2 in, 1 out]
            n163 = Set File Position(refnum=w270, from (0:start)=enum16{"start", "end", "current"}."end") -> ()  [unwired: 2 in, 2 out]
          }
          frame #4 {
          }
        }
        n164 = Wait (ms)(milliseconds to wait=u32 100) -> ()  [unwired: 1 out]
        "Status:" <- "Инициализация" ("Status:")
      }
      frame "TEC_Chars" {
        n165 = disable-structure shown="Disabled" {
          disable-tunnel: [w278 _] -> w277
          frame Disabled {
            n166 = while {
              tunnel: [w280] -> w278
              stop <- w279 stop-if-true
              n167 = stacked-sequence {
                tunnel: [_ _ w326 _] -> w280
                tunnel: [_ _ w324 _] -> w279
                frame #0 {
                  n168 = local write "Boolean 2"(FALSE) -> ()
                  n169 = stacked-sequence {
                    frame #0 {
                      # "Переключение в режим Омметра"
                      n170 = local read "4070_Rele_source"() -> (w286:enum16{"S2_Ch0", "S1_Ch2"})
                      n171 = case shown="\"S2_Ch0\", Default" w286 {
                        tunnel: [5.0 -5.0] -> w285
                        tunnel: ["0" "2"] -> w284
                        tunnel: [w287 w290] -> w283
                        frame "S2_Ch0", Default {
                          n172 = local read "Source_2_Vcc_out"() -> (w287:refnum<k15>)
                        }
                        frame "S1_Ch2" {
                          n173 = local read "Source_1_Vcc_out"() -> (w290:refnum<k15>)
                        }
                      }
                      n174 = call <instrlib>:"niDCPower Configure Voltage Level.vi"("voltage level"=w285, "channel name"=w284, "instrument handle"=w283) -> ()  [unwired: 7 in, 2 out]
                    }
                    frame #1 {
                      w293 = FALSE
                      # "Отключение стабилизации"
                      n175 = while {
                        tunnel: w293 -> [_]
                        stop <- w294 stop-if-true
                        n176 = local read "NoStab"() -> (w294:bool)
                      }
                      n177 = local write "ThRes_stabil"(w293) -> ()
                    }
                    frame #2 {
                      # "Перестановка in0 и in1 (+ и - у Пельтье)"
                      n178 = local read "Source_2_Vcc_out"() -> (w296:refnum<k15>)
                      n179 = call <instrlib>:"niDCPower Configure Voltage Level.vi"("voltage level"=-5.0, "channel name"="2", "instrument handle"=w296) -> ()  [unwired: 7 in, 2 out]
                    }
                    frame #3 {
                      # "Отключение пельтье"
                      n180 = local read "Source_1_Vcc_out"() -> (w298:refnum<k15>)
                      n181 = call <instrlib>:"niDCPower Configure Voltage Level.vi"("voltage level"=0.0, "channel name"="2", "instrument handle"=w298) -> ()  [unwired: 7 in, 2 out]
                    }
                    frame #4 {
                      n182 = Wait (ms)(milliseconds to wait="trelax") -> ()  [unwired: 1 out]
                    }
                  }
                  n183 = local write "Status:"("Выравнивание температуры" ("Status:")) -> ()
                }
                frame #1 {
                  w309 = T4 6.5 items=["3 1/2"=3.5, "4 1/2"=4.5, "5 1/2"=5.5, "6 1/2"=6.5, "7 1/2"=7.5] ("Resolution in Digits")
                  n184 = local write "Выполняется"(TRUE) -> ()
                  n185 = local read "4070_address"() -> (w308:refnum<k15>)
                  n186 = call-poly <instrlib>:"niDMM Config Measurement.vi"("Range"=-1.0 ("Configuration:Measurement Options:Max Frequency"), "Resolution in Digits"=w309, "Function"=niDMM_Function."2-wire Resistance" ("multimeter mode"), "instrument handle"=w308) -> ("instrument handle out"=w305:refnum<k15>)  [unwired: 6 in, 1 out]
                  n187 = for {
                    N: 2 -> [_]
                    tunnel: w305 -> [w315]
                    tunnel: [w314] -> w304
                    n188 = call <instrlib>:"niDMM Read.vi"("instrument handle"=w315) -> ("instrument handle out"=w314:refnum<k15>)  [unwired: 8 in, 2 out]
                  }
                  n189 = for {
                    N: 5 -> [_]
                    tunnel: w304 -> [w317]
                    tunnel: [w316] -> w307 mode=indexing
                    n190 = call <instrlib>:"niDMM Read.vi"("instrument handle"=w317) -> ("Measurement"=w316:dbl)  [unwired: 8 in, 2 out]
                    n191 = Wait (ms)(milliseconds to wait=u32 100) -> ()  [unwired: 1 out]
                  }
                  n192 = call-poly <vilib>:"Mean.vi"("X"=w307) -> ("mean"=→"Ro, Ом":dbl)  [unwired: 1 out]
                  n193 = local write "Status:"("Измерение сопротивления в отсутствии тока " ("Status:")) -> ()
                }
                frame #2 {
                  # "Подстройка тока\nдля пельтье"
                  # "При достижении 0V поменять\nполярность, поменяв направление\nтока с помощью реле"
                  n194 = Add(x="Начальное\nнапряжение TEC, В", y="Шаг напр\nдля TEC, В") -> (x+y=w319:dbl)
                  n195 = for {
                    N: "кол-во точек для TEC" -> [_]
                    tunnel: [w349] -> w321 mode=indexing
                    tunnel: [w348] -> w323 mode=indexing
                    tunnel: "Шаг напр\nдля TEC, В" -> [w345]
                    tunnel: [w344] -> w320 mode=indexing
                    shift-right: [w347] -> _
                    shift-left: w319 -> [w346]
                    i -> [w343]
                    # "R"
                    # "I"
                    # "V"
                    n196 = stacked-sequence {
                      seq-local: [w351 _ _] -> [_ w380 _]
                      tunnel: [_ w381 _] -> w348
                      tunnel: [_ _ w409] -> w349
                      tunnel: [_ w380 _] -> w347
                      tunnel: w346 -> [w353 _ _]
                      tunnel: w345 -> [w352 _ _]
                      tunnel: [w350 _ _] -> w344
                      frame #0 {
                        n197 = disable-structure shown="Enabled" {
                          disable-tunnel: w353 -> [w358 w377]
                          disable-tunnel: w352 -> [w357 w378]
                          disable-tunnel: [w356 w376] -> w351
                          disable-tunnel: [w355 w375] -> w350
                          frame Disabled {
                            n198 = local read "кол-во точек для TEC"() -> (w363:i32)
                            n199 = local read item#-1() -> (w360)
                            n200 = Divide(x=w363, y=2) -> (x/y=w361:dbl)
                            n201 = Less?(x=w361, y=w360) -> (x < y?=w359:bool)
                            n202 = case shown="False" w359 {
                              tunnel: [0.0 -5.0] -> w364
                              tunnel: w358 -> [w367 w373]
                              tunnel: w357 -> [w366 w372]
                              tunnel: [w365 w371] -> w356
                              tunnel: [w365 w369] -> w355
                              frame False {
                                n203 = Add(x=w367, y=w366) -> (x+y=w365:dbl)
                              }
                              frame True {
                                n204 = Subtract(x=w373, y=w372) -> (x-y=w371:dbl)
                                n205 = Multiply(x=-1.0, y=w371) -> (x*y=w369:dbl)
                              }
                            }
                          }
                          frame Enabled {
                            n206 = Subtract(x=w377, y=w378) -> (x-y=w376:dbl)
                            n207 = Multiply(x=-1.0, y=w376) -> (x*y=w375:dbl)
                          }
                        }
                        n208 = Wait (ms)(milliseconds to wait=u32 100) -> ()  [unwired: 1 out]
                      }
                      frame #1 {
                        n209 = case shown="\"S1_Ch2\", Default" "TEC_Source" {
                          tunnel: [w404 w406 w408] -> w383
                          tunnel: ["2" "0" "1"] -> w382
                          frame "S1_Ch2", Default {
                            n210 = local read "Source_1_Vcc_out"() -> (w404:refnum<k15>)
                          }
                          frame "S2_Ch0" {
                            n211 = local read "Source_2_Vcc_out"() -> (w406:refnum<k15>)
                          }
                          frame "S3_Ch1" {
                            n212 = local read "Source_3_Vcc_out"() -> (w408:refnum<k15>)
                          }
                        }
                        n213 = flat-sequence {
                          tunnel: [w392] -> w387
                          tunnel: [w389] -> w386
                          tunnel: w383 -> [w391]
                          tunnel: w382 -> [w389]
                          tunnel: w380 -> [w390]
                          tunnel: w387 -> [w393]
                          tunnel: w386 -> [w394]
                          tunnel: [w394] -> w385
                          tunnel: [w393] -> w384
                          tunnel: w385 -> [w399]
                          tunnel: w384 -> [w400]
                          tunnel: [w402] -> w381
                          frame #0 {
                            n214 = call <instrlib>:"niDCPower Configure Voltage Level.vi"("voltage level"=w390, "channel name"=w389, "instrument handle"=w391) -> ("instrument handle out"=w392:refnum<k15>)  [unwired: 7 in, 1 out]
                          }
                          frame #1 {
                            n215 = Wait (ms)(milliseconds to wait=u32 100) -> ()  [unwired: 1 out]
                          }
                          frame #2 {
                            w401 = T6 0 items=["Current", "Voltage"] ("measurement type")
                            n216 = call <instrlib>:"niDCPower Measure.vi"("measurement type"=w401, "channel name"=w399, "instrument handle"=w400) -> ("measurement"=w398:dbl)  [unwired: 6 in, 2 out]
                            n217 = Multiply(x=w398, y=1000.0) -> (x*y=w396:dbl)
                            n218 = Absolute Value(x=w396) -> (abs(x)=w402:dbl)
                            "TEC_current, mA" <- w402
                          }
                        }
                      }
                      frame #2 {
                        w414 = T4 6.5 items=["3 1/2"=3.5, "4 1/2"=4.5, "5 1/2"=5.5, "6 1/2"=6.5, "7 1/2"=7.5] ("Resolution in Digits")
                        # "Снятие показаний\nТерморезистора"
                        n219 = local read "4070_address"() -> (w413:refnum<k15>)
                        n220 = call-poly <instrlib>:"niDMM Config Measurement.vi"("Range"=-1.0 ("Configuration:Measurement Options:Max Frequency"), "Resolution in Digits"=w414, "Function"=niDMM_Function."2-wire Resistance" ("multimeter mode"), "instrument handle"=w413) -> ("instrument handle out"=w412:refnum<k15>)  [unwired: 6 in, 1 out]
                        n221 = for {
                          N: 10 -> [_]
                          tunnel: w412 -> [w418]
                          tunnel: [w417] -> w411 mode=indexing
                          n222 = call <instrlib>:"niDMM Read.vi"("instrument handle"=w418) -> ("Measurement"=w417:dbl)  [unwired: 8 in, 2 out]
                          n223 = Wait (ms)(milliseconds to wait=u32 20) -> ()  [unwired: 1 out]
                        }
                        n224 = call-poly <vilib>:"Mean.vi"("X"=w411) -> ("mean"=w409:dbl)  [unwired: 1 out]
                      }
                    }
                    n225 = Equal?(x=0, y=w343) -> (x = y?=w341:bool)
                    n226 = Select(t=u32 3000, s=w341, f="milliseconds to wait") -> (s? t:f=w340:u32)
                    n227 = Wait (ms)(milliseconds to wait=w340) -> ()  [unwired: 1 out]
                  }
                  n228 = local write "Status:"("Построение характеристики TEC" ("Status:")) -> ()
                  n229 = flat-sequence {
                    tunnel: [T1."TRes_Check(Idle)" ("Case")] -> w326
                    tunnel: w323 -> [w335]
                    tunnel: [TRUE] -> w324
                    tunnel: w321 -> [w333]
                    tunnel: w321 -> [w331]
                    tunnel: w320 -> [w330]
                    frame #0 {
                      # "Построение харак-ки TEC\nи опциональная запись"
                      n230 = Bundle(w335, w333) -> (→"RES(I_TEC) Graph":cluster{dbl[], dbl[]})  [unwired: 1 in]
                      n231 = Bundle(w330, w331) -> (→"RES(U_TEC) Graph":cluster{dbl[], dbl[]})  [unwired: 1 in]
                      n232 = local write "Выполняется"(FALSE) -> ()
                    }
                  }
                }
                frame #3 {
                  n233 = disable-structure shown="Disabled" {
                    frame Disabled {
                      # "Переключение в режим Вольтметра"
                      n234 = local read "4070_Rele_source"() -> (w422:enum16{"S2_Ch0", "S1_Ch2"})
                      n235 = case shown="\"S2_Ch0\", Default" w422 {
                        tunnel: [0.0 0.0] -> w425
                        tunnel: ["0" "2"] -> w424
                        tunnel: [w426 w429] -> w423
                        frame "S2_Ch0", Default {
                          n236 = local read "Source_2_Vcc_out"() -> (w426:refnum<k15>)
                        }
                        frame "S1_Ch2" {
                          n237 = local read "Source_1_Vcc_out"() -> (w429:refnum<k15>)
                        }
                      }
                      n238 = call <instrlib>:"niDCPower Configure Voltage Level.vi"("voltage level"=w425, "channel name"=w424, "instrument handle"=w423) -> ()  [unwired: 7 in, 2 out]
                    }
                    frame Enabled {
                    }
                  }
                  n239 = Wait (ms)(milliseconds to wait=u32 1000) -> ()  [unwired: 1 out]
                  n240 = local write "ThRes_stabil"(TRUE) -> ()
                }
              }
            }
          }
          frame Enabled {
          }
        }
      }
      frame "TRes_Check(Idle)" {
        n241 = flat-sequence {
          tunnel: [w456] -> w436
          tunnel: [w458] -> w435
          tunnel: w436 -> [w459]
          tunnel: w435 -> [w461]
          tunnel: [w460] -> w432
          tunnel: [w481] -> w434
          tunnel: w432 -> [w481]
          frame #0 {
            w446 = i16 3 ("width (-)")
            w440 = "\t"
            w453 = i16 3 ("width (-)")
            w454 = i16 3 ("width (-)")
            n242 = local read "refnum out"() -> (w458:refnum<file>)
            n243 = local read "Operating Current, mA"() -> (w439:dbl)
            n244 = local read "I_pd, uA"() -> (w437:dbl)
            n245 = local read "IPD(ext), mA"() -> (w452:dbl)
            n246 = Select(t="Облучение", s="Облучение!", f="") -> (s? t:f=w441:string)
            n247 = Get Date/Time In Seconds() -> (seconds since 1Jan1904=w450:timestamp)
            n248 = Format Date/Time String(time format string (%c)="%d  %H:%M:%S", seconds (now)=w450) -> (date/time string=w449:string)  [unwired: 1 in]
            n249 = Number To Fractional String(number=w439, width (-)=w454, precision (6)=w454) -> (F-format string=w448:string)  [unwired: 1 in]
            n250 = Number To Fractional String(number=w452, width (-)=w453, precision (6)=w453) -> (F-format string=w447:string)  [unwired: 1 in]
            n251 = Number To Fractional String(number=w437, width (-)=w446, precision (6)=w446) -> (F-format string=w445:string)  [unwired: 1 in]
            n252 = Greater?(x=w439, y="Порог типатиристора, мА") -> (0:w457:bool)
            n253 = Format Into String(initial string=w458, w449, w440, w448, w440, w447, w440, w445, w440, w441, w440) -> ()  [unwired: 2 in, 2 out]
            n254 = Or(x="SEL simulation", y=w457) -> (x .or. y?=w456:bool)
          }
          frame #1 {
            n255 = case shown="True" w459 {
              tunnel: ["" w466] -> w463
              tunnel: [T1."TRes_Check(Idle)" ("Case") w467] -> w460
              frame False {
              }
              frame True {
                n256 = stacked-sequence {
                  tunnel: [_ _ T1."TRes_Check(Idle)" ("Case")] -> w467
                  tunnel: [_ _ "!!!!"] -> w466
                  frame #0 {
                    n257 = local read "Source_1_Vcc_out"() -> (w469:refnum<k15>)
                    n258 = call <instrlib>:"niDCPower Configure Voltage Level.vi"("voltage level"=0.0, "channel name"="0", "instrument handle"=w469) -> ()  [unwired: 7 in, 2 out]
                  }
                  frame #1 {
                    n259 = Wait (ms)(milliseconds to wait="milliseconds to wait 2") -> ()  [unwired: 1 out]
                  }
                  frame #2 {
                    n260 = local read "accommodated voltage (out)"() -> (w473:dbl)
                    n261 = local read "Счетчик сбоев"() -> (w476:dbl)
                    n262 = local read "Source_1_Vcc_out"() -> (w474:refnum<k15>)
                    n263 = Increment(x=w476) -> (x+1=w477:dbl)
                    n264 = local write "Счетчик сбоев"(w477) -> ()
                    n265 = call <instrlib>:"niDCPower Configure Voltage Level.vi"("voltage level"=w473, "channel name"="0", "instrument handle"=w474) -> ()  [unwired: 7 in, 2 out]
                    n266 = local write "SEL simulation"(FALSE) -> ()
                  }
                }
              }
            }
            n267 = Format Into String(initial string=w461, w463, "\r\n") -> ()  [unwired: 2 in, 2 out]
          }
          frame #2 {
            n268 = Wait (ms)(milliseconds to wait=u32 250) -> ()  [unwired: 1 out]
          }
        }
        n269 = local write "Status:"("IDLE" ("Status:")) -> ()
      }
      frame "Characteristics" {
        n270 = disable-structure shown="Disabled" {
          disable-tunnel: [w484 _] -> w482
          frame Disabled {
            n271 = flat-sequence {
              tunnel: [w502] -> w495
              tunnel: [w506] -> w494
              tunnel: [w505] -> w493
              tunnel: [w504] -> w492
              tunnel: [w501] -> w491
              tunnel: [w499] -> w490
              tunnel: w495 -> [w736]
              tunnel: [w736] -> w489
              tunnel: w494 -> [w721]
              tunnel: [w721] -> w488
              tunnel: w493 -> [w738]
              tunnel: [w738] -> w487
              tunnel: w492 -> [w722]
              tunnel: [w722] -> w486
              tunnel: w491 -> [w737]
              tunnel: [w737] -> w485
              tunnel: w490 -> [w712]
              tunnel: [T1."TRes_Check(Idle)" ("Case")] -> w484
              tunnel: w489 -> [w739]
              tunnel: w488 -> [w759]
              tunnel: w487 -> [w758]
              tunnel: w486 -> [w756]
              tunnel: w485 -> [w753]
              frame #0 {
                n272 = local read "Отладка(F)/\n/Рабочий(T)"() -> (w496:bool)
                n273 = case shown="True" w496 {
                  frame False {
                  }
                  frame True {
                    n274 = while {
                      stop <- w498 stop-if-true
                      n275 = call "Save_dialogue_dose.vi"() -> ("output 1"=w497:dbl)  [unwired: 11 in]
                      n276 = Not Equal To 0?(x=w497) -> (x != 0?=w498:bool)
                    }
                  }
                }
              }
              frame #1 {
                # "Хар-ки:\nI_LD (V);\nOphir(I_LD);\nI_PD(I_LD);\nRcheck(I_LD)"
                n277 = Subtract(x="Начальный ток, мА", y="Шаг, мА") -> (x-y=w507:dbl)
                n278 = for {
                  N: "Кол-во точек" -> [_]
                  shift-right: [w516] -> _
                  shift-left: w507 -> [w518]
                  tunnel: [w516] -> w502 mode=indexing
                  tunnel: [w515] -> w506 mode=indexing
                  tunnel: [w514] -> w505 mode=indexing
                  tunnel: [w513] -> w504 mode=indexing
                  tunnel: [w511] -> w501 mode=indexing
                  tunnel: [w509] -> w499
                  i -> [w512]
                  # "ExtPD"
                  # "FV"
                  # "I_PD"
                  # "I_LD"
                  # "Ophir"
                  n279 = property on="Шаг, мА" class="DigNum (strict)"() -> ("Value"=w510:dbl)  [unwired: 2 in, 2 out]
                  n280 = Add(x=w518, y=w510) -> (x+y=w517:dbl)
                  n281 = stacked-sequence {
                    tunnel: w517 -> [_ w539 _ _ _ _ _ _ _]
                    tunnel: [_ w533 _ _ _ _ _ _ _] -> w516
                    tunnel: [_ _ _ _ _ w602 _ _ _] -> w515
                    tunnel: [_ _ _ _ _ _ w618 _ _] -> w514
                    tunnel: [_ _ _ _ w593 _ _ _ _] -> w513
                    tunnel: w512 -> [_ _ _ _ _ _ _ _ w655]
                    tunnel: [_ _ _ _ _ _ _ w631 _] -> w511
                    tunnel: [_ _ _ _ _ _ _ _ w654] -> w509
                    frame #0 {
                      n282 = disable-structure shown="Disabled" {
                        frame Disabled {
                          n283 = stacked-sequence {
                            frame #0 {
                              w519 = FALSE
                              # "Отключение стабилизации"
                              n284 = while {
                                tunnel: w519 -> [_]
                                stop <- w520 stop-if-true
                                n285 = local read "NoStab"() -> (w520:bool)
                              }
                              n286 = local write "ThRes_stabil"(w519) -> ()
                            }
                            frame #1 {
                              # "Переключение в режим Вольтметра"
                              n287 = local read "4070_Rele_source"() -> (w521:enum16{"S2_Ch0", "S1_Ch2"})
                              n288 = case shown="\"S2_Ch0\", Default" w521 {
                                tunnel: [0.0 0.0] -> w524
                                tunnel: ["0" "2"] -> w523
                                tunnel: [w525 w528] -> w522
                                frame "S2_Ch0", Default {
                                n289 = local read "Source_2_Vcc_out"() -> (w525:refnum<k15>)
                                }
                                frame "S1_Ch2" {
                                n290 = local read "Source_1_Vcc_out"() -> (w528:refnum<k15>)
                                }
                              }
                              n291 = call <instrlib>:"niDCPower Configure Voltage Level.vi"("voltage level"=w524, "channel name"=w523, "instrument handle"=w522) -> ()  [unwired: 7 in, 2 out]
                            }
                          }
                        }
                        frame Enabled {
                        }
                      }
                    }
                    frame #1 {
                      # "Подстройка тока\nлазерного диода"
                      n292 = local read "Source_1_Vcc_out"() -> (w540:refnum<k15>)
                      n293 = disable-structure shown="Enabled" {
                        disable-tunnel: "the lower limit for the voltage_LD" -> [w557 w563]
                        disable-tunnel: "Start voltage_LD" -> [w556 w564]
                        disable-tunnel: "the upper limit for the voltage_LD" -> [w555 w565]
                        disable-tunnel: w540 -> [w554 w562]
                        disable-tunnel: w539 -> [w553 w561]
                        disable-tunnel: "Res_LD" -> [w552 w560]
                        disable-tunnel: "0" -> [w551 w558]
                        disable-tunnel: "accuracy_LD" -> [w550 w568]
                        disable-tunnel: [w549 w567] -> w535
                        disable-tunnel: [w547 w566] -> w534
                        disable-tunnel: [w546 w559] -> w533
                        frame Disabled {
                          n294 = local read "4070_address"() -> (w548:refnum<k15>)
                          n295 = call "Set input current_ChAmmeter.vi"("the lower limit for the voltage"=w557, "accuracy (input)"=w550, "4070_address"=w548, "Start voltage"=w556, "the upper limit for the voltage"=w555, "instrument handle"=w554, "the optimum current(input)"=w553, "res(input)"=w552, "channel name"=w551) -> ("accommodated voltage (out)"=w549:dbl, "current value, mA"=w546:dbl, "the voltage drop across the resistor"=w547:dbl)  [unwired: 3 in, 1 out]
                        }
                        frame Enabled {
                          n296 = call "Set input current_ChSource.vi"("channel name"=w558, "res(input)"=w560, "the optimum current(input)"=w561, "accuracy (input)"=w568, "instrument handle"=w562, "the upper limit for the voltage"=w565, "Start voltage"=w564, "the lower limit for the voltage"=w563) -> ("current value, mA"=w559:dbl, "the voltage drop across the resistor"=w566:dbl, "accommodated voltage (out)"=w567:dbl)  [unwired: 1 out]
                        }
                      }
                      "Подстроенный ток, mA" <- w533
                      "accommodated voltage (out)" <- w535
                      "Volt_onRes" <- w534
                      n297 = local write "Status:"("Подстройка тока LD" ("Status:")) -> ()
                      n298 = Wait (ms)(milliseconds to wait=u32 100) -> ()  [unwired: 1 out]
                      n299 = Greater Or Equal?(x=w533, y=49.5) -> (x >= y?=→"Boolean":bool)
                    }
                    frame #2 {
                      # "and stab"
                      # "Resistance check"
                      n300 = flat-sequence {
                        frame #0 {
                          n301 = disable-structure shown="Disabled" {
                            frame Disabled {
                              # "Режим Омметра"
                              n302 = case shown="\"S2_Ch0\", Default" "4070_Rele_source" {
                                tunnel: [5.0 -5.0] -> w572
                                tunnel: ["0" "2"] -> w571
                                tunnel: [w574 w577] -> w570
                                frame "S2_Ch0", Default {
                                n303 = local read "Source_2_Vcc_out"() -> (w574:refnum<k15>)
                                }
                                frame "S1_Ch2" {
                                n304 = local read "Source_1_Vcc_out"() -> (w577:refnum<k15>)
                                }
                              }
                              n305 = call <instrlib>:"niDCPower Configure Voltage Level.vi"("voltage level"=w572, "channel name"=w571, "instrument handle"=w570) -> ()  [unwired: 7 in, 2 out]
                            }
                            frame Enabled {
                            }
                          }
                        }
                        frame #1 {
                          n306 = Wait (ms)(milliseconds to wait=u32 1000) -> ()  [unwired: 1 out]
                          "Num_hits" <- u64 0 ("Num_hits")
                        }
                        frame #2 {
                          n307 = local write "ThRes_stabil"(TRUE) -> ()
                        }
                        frame #3 {
                          n308 = local write "Count_hits?"(TRUE ("Acq_allow?")) -> ()
                          n309 = Wait (ms)(milliseconds to wait="tstab между точками, мс") -> ()  [unwired: 1 out]
                        }
                      }
                      n310 = local write "Status:"("Проверка и стабилизация сопротивления" ("Status:")) -> ()
                    }
                    frame #3 {
                      n311 = while {
                        tunnel: [u64 0] -> w586
                        tunnel: [FALSE ("Acq_allow?")] -> w585
                        stop <- w589 stop-if-true
                        n312 = local read "Num_hits"() -> (w591:u64)
                        n313 = Greater Or Equal?(x=w591, y="Num_hits_req") -> (x >= y?=w589:bool)
                      }
                      n314 = local write "Count_hits?"(w585) -> ()
                      n315 = local write "Num_hits"(w586) -> ()
                    }
                    frame #4 {
                      # "Forward\nVoltage\nmeasurement"
                      n316 = local read "Source_1_Vcc_out"() -> (w599:refnum<k15>)
                      n317 = local read "Volt_onRes"() -> (w592:dbl)
                      n318 = call <instrlib>:"niDCPower Measure Multiple.vi"("channel name"="0", "instrument handle"=w599) -> ("voltage measurements"=w597:dbl[])  [unwired: 6 in, 3 out]
                      n319 = Index Array(array=w597) -> (element=w595:dbl)  [unwired: 1 in]
                      n320 = Absolute Value(x=w592) -> (abs(x)=w594:dbl)
                      n321 = Absolute Value(x=w595) -> (abs(x)=w596:dbl)
                      n322 = Subtract(x=w596, y=w594) -> (x-y=w593:dbl)
                      "Forward Voltage, V" <- w593
                      n323 = local write "Status:"("Измерение прямого напряжения" ("Status:")) -> ()
                      n324 = Wait (ms)(milliseconds to wait=u32 100) -> ()  [unwired: 1 out]
                    }
                    frame #5 {
                      # "Ophir\nmeasurement"
                      n325 = property on="Ophir_address" class="Ref (strict)"() -> ("Value"=w604:refnum<k7>)  [unwired: 2 in, 2 out]
                      n326 = property on="hDevice" class="DigNum (strict)"() -> ("Value"=w603:i32)  [unwired: 2 in, 2 out]
                      n327 = invoke class="ICoLMMeasurement" method="GetData"(reference=w604, "hDevice"=w603, "channel"=0) -> ("arrayValue"=w611:variant)  [unwired: 5 in, 7 out]
                      n328 = local write "Status:"("Измерен. оптич. мощности" ("Status:")) -> ()
                      n329 = Variant To Data(type=dbl[] [], Variant=w611) -> (data=w608:dbl[])  [unwired: 1 in, 1 out]
                      n330 = Wait (ms)(milliseconds to wait=u32 200) -> ()  [unwired: 1 out]
                      n331 = Array Size(array=w608) -> (size(s)=w606:i32)
                      n332 = Decrement(x=w606) -> (x-1=w605:i32)
                      n333 = Index Array(array=w608, index=w605) -> (element=w607:dbl)
                      n334 = Multiply(x=1000.0, y=w607) -> (x*y=w602:dbl)
                      "Ophir, mW" <- w602
                    }
                    frame #6 {
                      w621 = T4 7.5 items=["3 1/2"=3.5, "4 1/2"=4.5, "5 1/2"=5.5, "6 1/2"=6.5, "7 1/2"=7.5] ("Resolution in Digits")
                      # "Inside I_PD\nmeasurements"
                      n335 = local read "4071(1)_adress"() -> (w622:refnum<k15>)
                      n336 = call-poly <instrlib>:"niDMM Config Measurement.vi"("Range"=-1.0 ("Configuration:Measurement Options:Max Frequency"), "Resolution in Digits"=w621, "Function"=niDMM_Function."DC Current" ("multimeter mode"), "instrument handle"=w622) -> ("instrument handle out"=w620:refnum<k15>)  [unwired: 6 in, 1 out]
                      n337 = for {
                        N: 5 -> [_]
                        tunnel: w620 -> [w629]
                        tunnel: [w626] -> w615 mode=indexing
                        n338 = call <instrlib>:"niDMM Read.vi"("instrument handle"=w629) -> ("Measurement"=w627:dbl)  [unwired: 8 in, 2 out]
                        n339 = Absolute Value(x=w627) -> (abs(x)=w626:dbl)
                        n340 = Wait (ms)(milliseconds to wait=u32 50) -> ()  [unwired: 1 out]
                      }
                      n341 = local write "Status:"("I_PD встроенного фотодиода" ("Status:")) -> ()
                      n342 = call-poly <vilib>:"Mean.vi"("X"=w615) -> ("mean"=w616:dbl)  [unwired: 1 out]
                      n343 = Multiply(x=w616, y=1000000.0) -> (x*y=w618:dbl)
                      "I_pd, uA" <- w618
                    }
                    frame #7 {
                      # "EXTERNAL I_PD\nmeasurements"
                      n344 = disable-structure shown="Enabled" {
                        disable-tunnel: [w634 w649] -> w631
                        disable-tunnel: [_ w649] -> w630
                        frame Disabled {
                          w641 = T4 6.5 items=["3 1/2"=3.5, "4 1/2"=4.5, "5 1/2"=5.5, "6 1/2"=6.5, "7 1/2"=7.5] ("Resolution in Digits")
                          n345 = local read "4071(2)_adress"() -> (w642:refnum<k15>)
                          n346 = call-poly <instrlib>:"niDMM Config Measurement.vi"("Range"=-1.0 ("Configuration:Measurement Options:Max Frequency"), "Resolution in Digits"=w641, "Function"=niDMM_Function."DC Current" ("multimeter mode"), "instrument handle"=w642) -> ("instrument handle out"=w640:refnum<k15>)  [unwired: 6 in, 1 out]
                          n347 = for {
                            N: 5 -> [_]
                            tunnel: w640 -> [w647]
                            tunnel: [w645] -> w638 mode=indexing
                            n348 = call <instrlib>:"niDMM Read.vi"("instrument handle"=w647) -> ("Measurement"=w645:dbl)  [unwired: 8 in, 2 out]
                            n349 = Wait (ms)(milliseconds to wait=u32 50) -> ()  [unwired: 1 out]
                          }
                          n350 = call-poly <vilib>:"Mean.vi"("X"=w638) -> ("mean"=w637:dbl)  [unwired: 1 out]
                          n351 = Absolute Value(x=w637) -> (abs(x)=w636:dbl)
                          n352 = Multiply(x=w636, y=1000.0) -> (x*y=w634:dbl)
                        }
                        frame Enabled {
                          n353 = local read "Source_2_Vcc_out"() -> (w653:refnum<k15>)
                          n354 = call <instrlib>:"niDCPower Measure Multiple.vi"("channel name"="1", "instrument handle"=w653) -> ("current measurements"=w651:dbl[])  [unwired: 6 in, 3 out]
                          n355 = Index Array(array=w651) -> (element=w648:dbl)  [unwired: 1 in]
                          n356 = Multiply(x=w648, y=1000.0) -> (x*y=w649:dbl)
                        }
                      }
                      "IPD(ext), mA" <- w630
                      n357 = local write "Status:"("I_PD внешнего фотодиода" ("Status:")) -> ()
                      n358 = Wait (ms)(milliseconds to wait=u32 200) -> ()  [unwired: 1 out]
                    }
                    frame #8 {
                      n359 = local read "Отладка(F)/\n/Рабочий(T)"() -> (w656:bool)
                      n360 = case shown="True" w656 {
                        tunnel: w655 -> [_ w675]
                        tunnel: [_ w657] -> w654
                        frame False {
                        }
                        frame True {
                          w665 = i16 3 ("width (-)")
                          w666 = i16 3 ("width (-)")
                          w668 = i16 3 ("width (-)")
                          w671 = i16 3 ("width (-)")
                          w674 = i16 3 ("width (-)")
                          # "Внешний ФД"
                          # "Офир"
                          n361 = local read "IPD(ext), mA"() -> (w659:dbl)
                          n362 = local read "Ophir, mW"() -> (w658:dbl)
                          n363 = local read "Forward Voltage, V"() -> (w670:dbl)
                          n364 = local read "Подстроенный ток, mA"() -> (w673:dbl)
                          n365 = local read "I_pd, uA"() -> (w667:dbl)
                          n366 = Equal To 0?(x=w675) -> (x = 0?=w663:bool)
                          n367 = Number To Fractional String(number=w673, width (-)=w674, precision (6)=w674) -> (F-format string=w672:string)  [unwired: 1 in]
                          n368 = Number To Fractional String(number=w670, width (-)=w671, precision (6)=w671) -> (F-format string=w669:string)  [unwired: 1 in]
                          n369 = Number To Fractional String(number=w659, width (-)=w668, precision (6)=w668) -> (F-format string=w660:string)  [unwired: 1 in]
                          n370 = Number To Fractional String(number=w667, width (-)=w666, precision (6)=w666) -> (F-format string=w661:string)  [unwired: 1 in]
                          n371 = Number To Fractional String(number=w658, width (-)=w665, precision (6)=w665) -> (F-format string=w662:string)  [unwired: 1 in]
                          n372 = case shown="True" w663 {
                            tunnel: ["" ("date/time string") w680] -> w657
                            tunnel: ["" w678] -> w664
                            frame False {
                            }
                            frame True {
                              w679 = i16 0 ("width (-)")
                              n373 = Get Date/Time In Seconds() -> (seconds since 1Jan1904=w682:timestamp)
                              n374 = Format Date/Time String(time format string (%c)="%d  %H:%M:%S", seconds (now)=w682) -> (date/time string=w680:string)  [unwired: 1 in]
                              n375 = Number To Fractional String(width (-)=w679, precision (6)=w679) -> (F-format string=w678:string)  [unwired: 2 in]
                            }
                          }
                          n376 = stacked-sequence {
                            tunnel: w657 -> [w689 w697 w704 _ w711]
                            tunnel: w664 -> [w688 w694 w702 _ w710]
                            tunnel: w672 -> [w686 w693 w701 _ w706]
                            tunnel: w669 -> [w684 _ _ _ _]
                            tunnel: w662 -> [_ w692 _ _ _]
                            tunnel: w661 -> [_ _ w699 _ _]
                            tunnel: w660 -> [_ _ _ _ w708]
                            frame #0 {
                              w685 = "\t"
                              n377 = Format Into String(w689, w685, "", w685, w688, w685, w686, w685, w684, "\r\n") -> ()  [unwired: 3 in, 2 out]
                            }
                            frame #1 {
                              w691 = "\t"
                              n378 = local read item#-1() -> (w696)
                              n379 = Format Into String(initial string=w696, w697, w691, "", w691, w694, w691, w693, w691, w692, "\r\n") -> ()  [unwired: 2 in, 2 out]
                            }
                            frame #2 {
                              w700 = "\t"
                              n380 = Format Into String(w704, w700, "", w700, w702, w700, w701, w700, w699, "\r\n") -> ()  [unwired: 3 in, 2 out]
                            }
                            frame #3 {
                            }
                            frame #4 {
                              w707 = "\t"
                              n381 = Format Into String(w711, w707, "", w707, w710, w707, w706, w707, w708, "\r\n") -> ()  [unwired: 3 in, 2 out]
                            }
                          }
                        }
                      }
                    }
                  }
                }
              }
              frame #2 {
                w718 = i16 3 ("width (-)")
                w724 = i16 3 ("width (-)")
                w726 = i16 3 ("width (-)")
                w729 = i16 3 ("width (-)")
                w731 = "" ("input 1")
                w716 = "\t"
                w734 = i16 3 ("width (-)")
                # "Рабочее напряжение"
                n382 = local read "Подстроенный ток, mA"() -> (w728:dbl)
                n383 = local read "Ophir, mW"() -> (w723:dbl)
                n384 = call "Find_ThresholdOphir_F4.vi"("Threshold Ophir"=5.0, "Current array"=w722, "Ophir array"=w721) -> ("Threshold Current"=w719:dbl)  [unwired: 8 in]
                n385 = call "Find_ThresholdOphir_F4.vi"("Threshold Ophir"=1.0, "Current array"=w736, "Ophir array"=w721) -> ("Threshold Current"=w733:dbl)  [unwired: 8 in]
                "Пороговый ток" <- w733
                n386 = local read "I_pd, uA"() -> (w717:dbl)
                n387 = Number To Fractional String(number=w719, width (-)=w726, precision (6)=w726) -> (F-format string=w725:string)  [unwired: 1 in]
                n388 = Number To Fractional String(number=w733, width (-)=w734, precision (6)=w734) -> (F-format string=w730:string)  [unwired: 1 in]
                n389 = Number To Fractional String(number=w717, width (-)=w718, precision (6)=w718) -> (F-format string=w714:string)  [unwired: 1 in]
                n390 = Number To Fractional String(number=w723, width (-)=w724, precision (6)=w724) -> (F-format string=w713:string)  [unwired: 1 in]
                n391 = Number To Fractional String(number=w728, width (-)=w729, precision (6)=w729) -> (F-format string=w727:string)  [unwired: 1 in]
                n392 = Format Into String(w712, w716, w731, w716, w731, w716, w730, w716, w727, w716, w725, w716, w714, w716, w713, "\r\n") -> (initial string=w732:refnum<file>)  [unwired: 2 in, 2 out]
              }
              frame #3 {
                n393 = property on="Boolean" class="Bool (strict)"() -> ("Value"=w748:bool)  [unwired: 2 in, 2 out]
                n394 = And(x=w748, y="Оставить в раб.\nрежиме") -> (x .and. y?=w749:bool)
                n395 = local read "Source_1_Vcc_out"() -> (w751:refnum<k15>)
                n396 = local read "Подстроенное напряжение\nстабилизации"() -> (w745:dbl)
                n397 = case shown="True" w749 {
                  tunnel: [0.0 ("voltage level") w764] -> w750
                  frame False {
                  }
                  frame True {
                    n398 = local read "accommodated voltage (out)"() -> (w764:dbl)
                  }
                }
                n399 = local read "Source_1_Vcc_out"() -> (w744:refnum<k15>)
                n400 = Bundle(w739, w759) -> (→"OP(I_LD) Graph":cluster{dbl[], dbl[]})  [unwired: 1 in]
                n401 = Bundle(w739, w758) -> (→"I_PD(I_LD) Graph":cluster{dbl[], dbl[]})  [unwired: 1 in]
                n402 = Bundle(w739, w756) -> (→"V2(I_LD) Graph":cluster{dbl[], dbl[]})  [unwired: 1 in]
                n403 = Bundle(w739, w753) -> (→"I_PD_Ext(I_LD) Graph":cluster{dbl[], dbl[]})  [unwired: 1 in]
                n404 = Add(x=w745, y=0.2) -> (x+y=w740:dbl)
                n405 = local write "Выполняется"(FALSE) -> ()
                n406 = Multiply(x=w740, y=-1.0) -> (x*y=w741:dbl)
                n407 = call <instrlib>:"niDCPower Configure Voltage Level.vi"("voltage level"=w741, "channel name"="2", "instrument handle"=w744) -> ()  [unwired: 7 in, 2 out]
                n408 = call <instrlib>:"niDCPower Configure Voltage Level.vi"("voltage level"=w750, "channel name"="0", "instrument handle"=w751) -> ()  [unwired: 7 in, 2 out]
              }
            }
            n409 = local write "Boolean 2"(FALSE) -> ()
          }
          frame Enabled {
          }
        }
      }
      frame "Bias" {
        n410 = local write "Boolean 2"(FALSE) -> ()
        n411 = stacked-sequence {
          tunnel: [_ _ _ _ _ w832] -> w765
          frame #0 {
            n412 = disable-structure shown="Disabled" {
              frame Disabled {
                w768 = FALSE
                n413 = while {
                  tunnel: w768 -> [_]
                  stop <- w769 stop-if-true
                  n414 = local read "NoStab"() -> (w769:bool)
                }
                n415 = local write "ThRes_stabil"(w768) -> ()
              }
              frame Enabled {
              }
            }
            n416 = local write "Num_hits"(0) -> ()
          }
          frame #1 {
            n417 = disable-structure shown="Disabled" {
              frame Disabled {
                # "Переключение в режим Вольтметра"
                n418 = local read "4070_Rele_source"() -> (w770:enum16{"S2_Ch0", "S1_Ch2"})
                n419 = case shown="\"S2_Ch0\", Default" w770 {
                  tunnel: [0.0 0.0] -> w773
                  tunnel: ["0" "2"] -> w772
                  tunnel: [w774 w777] -> w771
                  frame "S2_Ch0", Default {
                    n420 = local read "Source_2_Vcc_out"() -> (w774:refnum<k15>)
                  }
                  frame "S1_Ch2" {
                    n421 = local read "Source_1_Vcc_out"() -> (w777:refnum<k15>)
                  }
                }
                n422 = call <instrlib>:"niDCPower Configure Voltage Level.vi"("voltage level"=w773, "channel name"=w772, "instrument handle"=w771) -> ()  [unwired: 7 in, 2 out]
              }
              frame Enabled {
              }
            }
          }
          frame #2 {
            n423 = local read "the upper limit for the voltage_LD"() -> (w786:dbl)
            n424 = local read "the lower limit for the voltage_LD"() -> (w788:dbl)
            n425 = local read "Source_1_Vcc_out"() -> (w785:refnum<k15>)
            n426 = local read "Start voltage_LD"() -> (w787:dbl)
            n427 = local read "accuracy_LD"() -> (w782:dbl)
            n428 = local read "Res_LD"() -> (w784:dbl)
            n429 = disable-structure shown="Enabled" {
              disable-tunnel: "Desirable Operating current, mA" -> [w800 w806]
              disable-tunnel: [w799 w807] -> w780
              disable-tunnel: w788 -> [w798 w810]
              disable-tunnel: w787 -> [w797 w801]
              disable-tunnel: w786 -> [w796 w802]
              disable-tunnel: w785 -> [w795 w803]
              disable-tunnel: w784 -> [w794 w805]
              disable-tunnel: "0" ("channel name") -> [w793 w804]
              disable-tunnel: w782 -> [w792 w809]
              disable-tunnel: [w791 w808] -> w781
              frame Disabled {
                n430 = local read "4070_address"() -> (w790:refnum<k15>)
                n431 = call "Set input current_ChAmmeter.vi"("the lower limit for the voltage"=w798, "accuracy (input)"=w792, "4070_address"=w790, "Start voltage"=w797, "the upper limit for the voltage"=w796, "instrument handle"=w795, "the optimum current(input)"=w800, "res(input)"=w794, "channel name"=w793) -> ("accommodated voltage (out)"=w791:dbl, "current value, mA"=w799:dbl)  [unwired: 3 in, 2 out]
              }
              frame Enabled {
                n432 = call "Set input current_ChSource.vi"("channel name"=w804, "res(input)"=w805, "the optimum current(input)"=w806, "accuracy (input)"=w809, "instrument handle"=w803, "the upper limit for the voltage"=w802, "Start voltage"=w801, "the lower limit for the voltage"=w810) -> ("current value, mA"=w807:dbl, "accommodated voltage (out)"=w808:dbl)  [unwired: 2 out]
              }
            }
            "Operating Current, mA" <- w780
            n433 = local write "Подстроенный ток, mA"(w780) -> ()
            n434 = local write "accommodated voltage (out)"(w781) -> ()
          }
          frame #3 {
            n435 = local read "+ V TEC для новой точки"() -> (w815:dbl)
            n436 = local read "Подстроенное напряжение\nстабилизации"() -> (w813:dbl)
            n437 = local read "Source_1_Vcc_out"() -> (w819:refnum<k15>)
            n438 = Multiply(x=w815, y=2.0) -> (x*y=w812:dbl)
            n439 = Add(x=w812, y=w813) -> (x+y=w811:dbl)
            n440 = Multiply(x=w811, y=-1.0) -> (x*y=w816:dbl)
            n441 = call <instrlib>:"niDCPower Configure Voltage Level.vi"("voltage level"=w816, "channel name"="2", "instrument handle"=w819) -> ()  [unwired: 7 in, 2 out]
          }
          frame #4 {
            n442 = disable-structure shown="Enabled" {
              frame Disabled {
                # "Переключение в режим Омметра"
                n443 = local read "4070_Rele_source"() -> (w825:enum16{"S2_Ch0", "S1_Ch2"})
                n444 = case shown="\"S2_Ch0\", Default" w825 {
                  tunnel: [5.0 -5.0] -> w824
                  tunnel: ["0" "2"] -> w823
                  tunnel: [w826 w829] -> w822
                  frame "S2_Ch0", Default {
                    n445 = local read "Source_2_Vcc_out"() -> (w826:refnum<k15>)
                  }
                  frame "S1_Ch2" {
                    n446 = local read "Source_1_Vcc_out"() -> (w829:refnum<k15>)
                  }
                }
                n447 = call <instrlib>:"niDCPower Configure Voltage Level.vi"("voltage level"=w824, "channel name"=w823, "instrument handle"=w822) -> ()  [unwired: 7 in, 2 out]
              }
              frame Enabled {
              }
            }
            n448 = local write "Выполняется"(FALSE) -> ()
            n449 = local write "ThRes_stabil"(TRUE) -> ()
          }
          frame #5 {
            n450 = flat-sequence {
              tunnel: [T1."TRes_Check(Idle)" ("Case")] -> w832
              frame #0 {
                n451 = Wait (ms)(milliseconds to wait=u32 3000) -> ()  [unwired: 1 out]
              }
              frame #1 {
                n452 = disable-structure shown="Enabled" {
                  disable-tunnel: [w835 w847] -> w834
                  frame Disabled {
                    n453 = local read "Operating Current, mA"() -> (w838:dbl)
                    n454 = Greater Or Equal?(x=w838, y=45.0) -> (x >= y?=w836:bool)
                    n455 = disable-structure shown="Enabled" {
                      disable-tunnel: w836 -> [w840 w846]
                      disable-tunnel: [w839 w846] -> w835
                      frame Disabled {
                        n456 = case shown="True" w840 {
                          tunnel: [FALSE w842] -> w839
                          frame False {
                          }
                          frame True {
                            n457 = Two Button Dialog(message="Ну шо, облучаем?", 1:"Нет" ("F button name (\"Cancel\")"), 2:"Да" ("T button name (\"OK\")")) -> (T button?=w842:bool)
                          }
                        }
                      }
                      frame Enabled {
                      }
                    }
                  }
                  frame Enabled {
                    n458 = while {
                      tunnel: [w848] -> w847
                      stop <- w848 stop-if-true
                      n459 = local read "Стабилизировано"() -> (w848:bool)
                    }
                  }
                }
                "Готовы облучать" <- w834
              }
              frame #2 {
                n460 = local write "Num_hits_req"(u64 0 ("Num_hits_req")) -> ()
              }
            }
          }
        }
      }
      frame "Quit" {
        w852 = FALSE
        n461 = local write "Status:"("Выход" ("Status:")) -> ()
        n462 = local write "Num_hits"(u64 0 ("Num_hits")) -> ()
        n463 = local write "stop"(w852) -> ()
        n464 = local write "Power Enable"(w852) -> ()
        n465 = local write "Прервать"(w852) -> ()
        n466 = local write "Count_hits?"(w852) -> ()
      }
    }
  }
  n467 = while {
    tunnel: w9 -> [w857]
    stop <- FALSE stop-if-true
    n468 = event shown="[0] \"stop\": Value Change" {
      selector: _ -> [_ _ _ _]
      dyn-events: _ -> [_ _ _ _]
      timeout: _ -> [_ _ _ _]
      tunnel: w857 -> [_ _ _ _]
      event "stop": Value Change {
        # "Работает, зараза, через раз"
        n469 = event-data() -> ()  [unwired: 1 in, 6 out]
        n470 = flat-sequence {
          frame #0 {
            n471 = local write "Case"(T1."Quit" ("Case")) -> ()
          }
          frame #1 {
            n472 = local write "stop"(FALSE) -> ()
            "Прервать" <- TRUE
          }
        }
      }
      event "Раб. режим LD": Value Change {
        n473 = event-data() -> ()  [unwired: 1 in, 6 out]
        n474 = flat-sequence {
          frame #0 {
            n475 = local write "Раб. режим LD"(FALSE) -> ()
            n476 = local write "Case"(T1."Bias" ("Case")) -> ()
          }
          frame #1 {
            n477 = local write "Выполняется"(TRUE) -> ()
          }
        }
      }
      event "Хар-ка TEC": Value Change {
        n478 = event-data() -> ()  [unwired: 1 in, 6 out]
        n479 = flat-sequence {
          frame #0 {
            n480 = local write "Хар-ка TEC"(FALSE) -> ()
            n481 = local write "Case"(T1."TEC_Chars" ("Case")) -> ()
          }
          frame #1 {
            n482 = local write "Выполняется"(TRUE) -> ()
          }
        }
      }
      event "Хар-ки от I_LD": Value Change {
        n483 = event-data() -> ()  [unwired: 1 in, 6 out]
        n484 = flat-sequence {
          frame #0 {
            n485 = local write "Хар-ки от I_LD"(FALSE) -> ()
            n486 = local write "Case"(T1."Characteristics" ("Case")) -> ()
          }
          frame #1 {
            n487 = local write "Выполняется"(TRUE) -> ()
          }
        }
      }
    }
  }
  n488 = while {
    tunnel: w8 -> [w871]
    tunnel: w7 -> [w872]
    stop <- FALSE stop-if-true
    w874 = T1."Initialization"  # Case
    n489 = disable-structure shown="Enabled" {
      frame Disabled {
        n490 = local read "Выполняется"() -> (w876:bool)
        n491 = Compound Arithmetic op=OR(w876) -> ()  [unwired: 1 in, 1 out]
      }
      frame Enabled {
      }
    }
    n492 = local read "Case"() -> (w873:T1)
    n493 = Equal?(x=w873, y=w874) -> (x = y?=w870:bool)
    n494 = case shown="False" w870 {
      tunnel: w872 -> [w878 _]
      tunnel: w871 -> [w877 _]
      frame False {
        n495 = stacked-sequence {
          tunnel: w878 -> [w881 w916 _ _ _]
          tunnel: w877 -> [w880 w915 _ _ _]
          frame #0 {
            n496 = local read "Power Enable"() -> (w879:bool)
            n497 = call <instrlib>:"niDCPower Configure Output Enabled.vi"("output enabled"=w879, "channel name"="0,1,2", "instrument handle"=w881) -> ()  [unwired: 7 in, 2 out]
            n498 = call <instrlib>:"niDCPower Configure Output Enabled.vi"("output enabled"=w879, "channel name"="0,1,2", "instrument handle"=w880) -> ()  [unwired: 7 in, 2 out]
          }
          frame #1 {
            w895 = "1"
            w899 = 1000.0 ("y")
            w906 = "0" ("channel name")
            n499 = Divide(x="Предел тока ТЕС, мА", y=1000.0) -> (x/y=w909:dbl)
            n500 = call <instrlib>:"niDCPower Configure Current Limit.vi"("current limit"=w909, "channel name"="2", "instrument handle"=w916) -> ("instrument handle out"=w888:refnum<k15>)  [unwired: 7 in, 1 out]
            n501 = call <instrlib>:"niDCPower Configure Current Limit.vi"("current limit"=w909, "channel name"="0", "instrument handle"=w915) -> ("instrument handle out"=w902:refnum<k15>)  [unwired: 7 in, 1 out]
            n502 = Divide(x="Предел тока LD, мА", y=w899) -> (x/y=w910:dbl)
            n503 = Divide(x="Предел тока PDext, мА", y=w899) -> (x/y=w901:dbl)
            n504 = call <instrlib>:"niDCPower Configure Current Limit.vi"("current limit"=w901, "channel name"=w895, "instrument handle"=w902) -> ("instrument handle out"=w894:refnum<k15>)  [unwired: 7 in, 1 out]
            n505 = call <instrlib>:"niDCPower Measure Multiple.vi"("channel name"="2", "instrument handle"=w888) -> ("current measurements"=w891:dbl[])  [unwired: 6 in, 3 out]
            n506 = call <instrlib>:"niDCPower Configure Current Limit.vi"("current limit"=w910, "channel name"=w906, "instrument handle"=w888) -> ("instrument handle out"=w907:refnum<k15>)  [unwired: 7 in, 1 out]
            n507 = call <instrlib>:"niDCPower Measure Multiple.vi"("channel name"=w895, "instrument handle"=w894) -> ("current measurements"=w896:dbl[])  [unwired: 6 in, 3 out]
            n508 = Index Array(array=w891) -> (element=w890:dbl)  [unwired: 1 in]
            n509 = call <instrlib>:"niDCPower Measure Multiple.vi"("channel name"=w906, "instrument handle"=w907) -> ("current measurements"=w905:dbl[])  [unwired: 6 in, 3 out]
            n510 = Multiply(x=w890, y=1000.0) -> (x*y=w892:dbl)
            n511 = Index Array(array=w896) -> (element=w897:dbl)  [unwired: 1 in]
            n512 = Absolute Value(x=w892) -> (abs(x)=w886:dbl)
            n513 = Index Array(array=w905) -> (element=w904:dbl)  [unwired: 1 in]
            n514 = Multiply(x=w897, y=1000.0) -> (x*y=w893:dbl)
            n515 = local write "TEC_current, mA"(w886) -> ()
            n516 = Absolute Value(x=w893) -> (abs(x)=w884:dbl)
            "ExtPhotodiode Current" <- w884
            n517 = Multiply(x=w904, y=1000.0) -> (x*y=w885:dbl)
            "Operating Current" <- w885
            n518 = local write "Operating Current, mA"(w885) -> ()
            n519 = local write "IPD(ext), mA"(w884) -> ()
          }
          frame #2 {
            n520 = Wait (ms)(milliseconds to wait=u32 100) -> ()  [unwired: 1 out]
          }
          frame #3 {
            n521 = local read "Source_2_Vcc_out"() -> (w922:refnum<k15>)
            n522 = Select(t=0.0, s="Нагрев", f=-5.0) -> (s? t:f=w920:dbl)
            n523 = call <instrlib>:"niDCPower Configure Voltage Level.vi"("voltage level"=w920, "channel name"="2", "instrument handle"=w922) -> ()  [unwired: 7 in, 2 out]
          }
          frame #4 {
            w928 = T4 6.5 items=["3 1/2"=3.5, "4 1/2"=4.5, "5 1/2"=5.5, "6 1/2"=6.5, "7 1/2"=7.5] ("Resolution in Digits")
            n524 = local read "4071(1)_adress"() -> (w927:refnum<k15>)
            n525 = call-poly <instrlib>:"niDMM Config Measurement.vi"("Range"=-1.0 ("Configuration:Measurement Options:Max Frequency"), "Resolution in Digits"=w928, "Function"=niDMM_Function."DC Current" ("multimeter mode"), "instrument handle"=w927) -> ("instrument handle out"=w929:refnum<k15>)  [unwired: 6 in, 1 out]
            n526 = for {
              N: 2 -> [_]
              tunnel: w929 -> [w936]
              tunnel: [w935] -> w931 mode=indexing
              n527 = call <instrlib>:"niDMM Read.vi"("instrument handle"=w936) -> ("Measurement"=w935:dbl)  [unwired: 8 in, 2 out]
            }
            n528 = call-poly <vilib>:"Mean.vi"("X"=w931) -> ("mean"=w932:dbl)  [unwired: 1 out]
            n529 = Absolute Value(x=w932) -> (abs(x)=w933:dbl)
            n530 = Multiply(x=w933, y=1000000.0) -> (x*y=w924:dbl)
            "Monitor current, uA" <- w924
            n531 = local write "I_pd, uA"(w924) -> ()
          }
        }
      }
      frame True {
        n532 = Wait (ms)(milliseconds to wait=u32 20) -> ()  [unwired: 1 out]
      }
    }
  }
  n533 = while {
    tunnel: w7 -> [w939]
    tunnel: w8 -> [w938]
    stop <- FALSE stop-if-true
    n534 = local read "stop"() -> (w940:bool)
    n535 = case shown="False" w940 {
      tunnel: w939 -> [_ w943]
      tunnel: w938 -> [_ w942]
      frame False {
      }
      frame True {
        n536 = stacked-sequence {
          tunnel: w943 -> [_ _ _ _ w950 _]
          tunnel: w942 -> [_ _ _ _ w949 _]
          frame #0 {
            w944 = T1."Initialization"  # Case
            n537 = local write "Case"(w944) -> ()
          }
          frame #1 {
            # "Закрытие логов"
            n538 = local read "refnum out"() -> (w945:refnum<file>)
            n539 = Format Into String(initial string=w945, "\r\n") -> (resulting string=w947:refnum<file>)  [unwired: 2 in, 1 out]
            n540 = Close File(refnum=w947) -> ()  [unwired: 1 in, 2 out]
          }
          frame #2 {
            # "Выключение Офира"
          }
          frame #3 {
            w948 = FALSE
            n541 = local write "Раб. режим LD"(w948) -> ()
            n542 = local write "Хар-ки от I_LD"(w948) -> ()
            n543 = local write "Power Enable"(w948) -> ()
            n544 = local write "Хар-ка TEC"(w948) -> ()
          }
          frame #4 {
            w953 = "0,1,2" ("channel name")
            w958 = "0,1,2" ("channel name")
            n545 = call <instrlib>:"niDCPower Configure Voltage Level.vi"("voltage level"=0.0, "channel name"=w958, "instrument handle"=w950) -> ("instrument handle out"=w957:refnum<k15>)  [unwired: 7 in, 1 out]
            n546 = call <instrlib>:"niDCPower Configure Voltage Level.vi"("voltage level"=0.0, "channel name"=w953, "instrument handle"=w949) -> ("instrument handle out"=w954:refnum<k15>)  [unwired: 7 in, 1 out]
            n547 = call <instrlib>:"niDCPower Configure Output Enabled.vi"("output enabled"=FALSE, "channel name"=w958, "instrument handle"=w957) -> ("instrument handle out"=w956:refnum<k15>)  [unwired: 7 in, 1 out]
            n548 = call <instrlib>:"niDCPower Configure Output Enabled.vi"("output enabled"=FALSE, "channel name"=w953, "instrument handle"=w954) -> ("instrument handle out"=w955:refnum<k15>)  [unwired: 7 in, 1 out]
            n549 = call <instrlib>:"niDCPower Close.vi"("instrument handle"=w956) -> ()  [unwired: 10 in, 1 out]
            n550 = call <instrlib>:"niDCPower Close.vi"("instrument handle"=w955) -> ()  [unwired: 10 in, 1 out]
          }
          frame #5 {
            n551 = Stop(stop? (T)=TRUE) -> ()
          }
        }
      }
    }
  }
  n552 = disable-structure shown="Disabled" {
    frame Disabled {
      n553 = local read "4070_address"() -> (w965:refnum<k15>)
      n554 = local read "TEC_Source"() -> (w962:enum16{"S1_Ch2", "S2_Ch0", "S3_Ch1"})
      n555 = case shown="\"S3_Ch1\"" w962 {
        tunnel: [w975 w977 w979] -> w964
        tunnel: ["2" "0" "1"] -> w963
        frame "S1_Ch2", Default {
          n556 = local read "Source_1_Vcc_out"() -> (w975:refnum<k15>)
        }
        frame "S2_Ch0" {
          n557 = local read "Source_2_Vcc_out"() -> (w977:refnum<k15>)
        }
        frame "S3_Ch1" {
          n558 = local read "Source_3_Vcc_out"() -> (w979:refnum<k15>)
        }
      }
      n559 = call "Res_stabiliz.vi"("Точность ThRes"="Точность ThRes", "Up_Volt_limit"="the upper limit for the voltage", "Optimum ThRes"="Optimum ThRes", "Low_Volt_limit"="the lower limit for the voltage", "TEC_Source"=w964, "4070_address"=w965, "channel name"=w963) -> ("Подстроенное напряжение"=→"Подстроенное напряжение\nстабилизации":dbl, "ThRes value"=→"ThRes value":dbl, "thRes_adj"=w973:dbl, "Start Voltage"=w966:dbl)  [unwired: 1 out]
      n560 = local write "Сопротивление терморез-ра"(w973) -> ()
    }
    frame Enabled {
    }
  }
  n561 = disable-structure shown="Disabled" {
    frame Disabled {
      w985 = T4 6.5 items=["3 1/2"=3.5, "4 1/2"=4.5, "5 1/2"=5.5, "6 1/2"=6.5, "7 1/2"=7.5] ("Resolution in Digits")
      n562 = local read "4070_address"() -> (w984:refnum<k15>)
      n563 = call-poly <instrlib>:"niDMM Config Measurement.vi"("Range"=-1.0 ("Configuration:Measurement Options:Max Frequency"), "Resolution in Digits"=w985, "Function"=niDMM_Function."2-wire Resistance" ("multimeter mode"), "instrument handle"=w984) -> ("instrument handle out"=w983:refnum<k15>)  [unwired: 6 in, 1 out]
      n564 = for {
        N: 3 -> [_]
        tunnel: w983 -> [w989]
        tunnel: [w988] -> w982 mode=indexing
        n565 = call <instrlib>:"niDMM Read.vi"("instrument handle"=w989) -> ("Measurement"=w988:dbl)  [unwired: 8 in, 2 out]
        n566 = Wait (ms)(milliseconds to wait=u32 50) -> ()  [unwired: 1 out]
      }
      n567 = call-poly <vilib>:"Mean.vi"("X"=w982) -> ("mean"=→"Сопротивление терморез-ра":dbl)  [unwired: 1 out]
    }
    frame Enabled {
    }
  }
  n568 = local write "Нагрев"(FALSE ("Нагрев")) -> ()
  n569 = disable-structure shown="Enabled" {
    frame Disabled {
      # "Есть в инициализации"
      # "Для измерения Сопротивления"
      # "Поменять in0/in1 для ТЕС"
      n570 = local read "Source_2_Vcc_out"() -> (w996:refnum<k15>)
      n571 = local read "4070_Rele_source"() -> (w991:enum16{"S2_Ch0", "S1_Ch2"})
      n572 = call <instrlib>:"niDCPower Configure Voltage Level.vi"("voltage level"=-5.0, "channel name"="2", "instrument handle"=w996) -> ()  [unwired: 7 in, 2 out]
      n573 = case shown="\"S1_Ch2\"" w991 {
        tunnel: [5.0 -5.0] -> w992
        tunnel: ["0" "2"] -> w993
        tunnel: [w998 w1001] -> w994
        frame "S2_Ch0", Default {
          n574 = local read "Source_2_Vcc_out"() -> (w998:refnum<k15>)
        }
        frame "S1_Ch2" {
          n575 = local read "Source_1_Vcc_out"() -> (w1001:refnum<k15>)
        }
      }
      n576 = call <instrlib>:"niDCPower Configure Voltage Level.vi"("voltage level"=w992, "channel name"=w993, "instrument handle"=w994) -> ()  [unwired: 7 in, 2 out]
    }
    frame Enabled {
    }
  }
  "Выполняется" <- w4
